vi "运维调试_质控单元.vi"() -> ()   [LabVIEW 2016, in "质控单元.lvlib"]
uses:
  <vilib>/Utility/miscctls.llb/LVPointTypeDef.ctl
  <vilib>/Analysis/6fits.llb/Curve Fitting Criteria.ctl
  <vilib>/Plasmionique/MB Master/MB_Master_Serial/MB_Master_Serial.lvclass
  D:/Program Files (x86)/National Instruments/LabVIEW 2016/vi.lib/Plasmionique/MB Master/MB_Master/MB_Master.lvclass
  <vilib>/Utility/config.llb/Write Key (I32).vi
  <vilib>/Utility/config.llb/Write Key (Double).vi
  <vilib>/Utility/config.llb/Write Key (Boolean).vi
  <vilib>/Utility/config.llb/Write Key (U32).vi
  <vilib>/Utility/config.llb/Read Key (I32).vi
  <vilib>/Utility/config.llb/Read Key (Double).vi
  <vilib>/Utility/config.llb/Read Key (Boolean).vi
  <vilib>/Utility/config.llb/Read Key (U32).vi
  <vilib>/Plasmionique/MB Master/MB Master.lvlib
  <vilib>/ptbypt/NI_PtbyPt.lvlib
  <vilib>/Utility/config.llb/NI_LVConfig.lvlib
  <vilib>/Analysis/NI_AALPro.lvlib
panel:
  out "COM口":string
  in  "总磷模块选择":enum32{"氨氮总磷", "总氮总磷"}(ring)=enum."总氮总磷"
  out "质控流程中":bool
  out "CODMn质控中断报警":bool
  out "总磷质控中断报警":bool
  out "总氮质控中断报警":bool
  out "氨氮质控中断报警":bool
  in  "报警清除":bool
  in  "CODMn量程选择":enum32{"H", "L", "AUTO"}(ring)
  in  "CODMn加标回收启动":bool
  in  "总磷总氮加标回收启动":bool
  in  "氨氮加标回收启动":bool
  in  "总磷量程选择":enum32{"H", "L", "AUTO"}(ring)=enum."AUTO"
  in  "总氮量程选择":enum32{"H", "L", "AUTO"}(ring)=enum."AUTO"
  in  "氨氮量程选择":enum32{"H", "L", "AUTO"}(ring)=enum."AUTO"
  out "COD超时报警":bool
  out "总磷总氮超时报警":bool
  out "氨氮进样超时报警":bool
  out "簇":T1
  out "通讯指示灯3":bool
  out "通讯指示灯2":bool
  out "通讯指示灯1":bool
  in  "CODMn":bool
  in  "总磷总氮":bool
  in  "氨氮":bool
  in  "枚举":enum16{"柱塞泵1", "柱塞泵2", "柱塞泵3"}(ring)
  in  "启用":bool
  in  "B 3":dbl caption="B3"
  in  "K 3":dbl caption="K3"
  in  "B 2":dbl caption="B2"
  in  "K 2":dbl caption="K2"
  in  "B":dbl caption="B1"
  in  "K":dbl caption="K1"
  out "r^2":dbl format="%_6g"
  out "拟合方程":string
  in  "实际体积 5":dbl
  in  "标准体积 5":dbl
  in  "实际体积 4":dbl
  in  "标准体积 4":dbl
  in  "实际体积 3":dbl
  in  "实际体积 2":dbl
  in  "实际体积 1":dbl
  in  "标准体积 3":dbl
  in  "标准体积 2":dbl
  in  "标准体积 1":dbl
  in  "读取":bool
  in  "柱塞泵3":bool
  in  "柱塞泵2":bool
  in  "柱塞泵1":bool
  in  "注出体积选择":u16(ring) items=["0.1mL", "0.3mL", "0.5mL", "0.8mL", "1.0mL"]
  out "Serial Config":T2={"baud rate (bps)"=115200, "stop bits"=10, "parity"=0, "flow control"=0, "timeout"=100, "retries"=1} {"stop bits" items=["1.0"=10, "1.5"=15, "2.0"=20]; "parity" items=["None", "Odd", "Even", "Mark", "Space"]; "flow control" items=["None", "XON/XOFF", "RTS/CTS", "XON/XOFF & RTS/CTS", "DTR/DSR", "XON/XOFF & DTR/DSR"]}
  out "VISA Resource":refnum<visa-resource-name>="COM8"
  in  "背隙补偿步数 3":i32 min=0 max=2000
  in  "背隙补偿步数 2":i32 min=0 max=2000
  in  "写入":bool
  in  "背隙补偿步数":i32 min=0 max=2000
  out "启动模块":T3
  out "COD传感器故障报警":bool
  in  "总氮停止":bool
  in  "总氮排液":bool
  in  "总氮调试":bool
  out "总氮加标回收率":dbl caption="加标回收率" format="%.2f"
  out "总氮加标体积":dbl caption="加标体积" format="%.3f"
  out "总氮母液浓度":dbl caption="加标母液浓度" format="%.3f"
  out "总氮加标水杯定容体积":dbl caption="加标水杯定容体积" format="%.2f"
  out "总氮加标后水样浓度":dbl caption="加标后水样浓度" format="%.3f"
  out "总氮加标前水样浓度":dbl caption="加标前水样浓度" format="%.3f"
  out "总氮检出限":dbl caption="检出限" format="%.3f"
  out "总氮量程":dbl caption="量程" format="%.2f"
  out "总氮状态":u16(ring) caption="状态" items=["待机", "润洗", "进样", "等待取液", "排液"]
  in  "返回":bool
  in  "查看":bool
  out "直接启动":bool
  out "常规启动":bool
  out "总磷总氮传感器故障报警":bool
  out "氨氮传感器故障报警":bool
  out "columns":string[](array[string])
  out "data":T4
  out "COD平行样测完标志":bool
  out "氨氮总磷平行样测完标志":bool
  out "输出簇 2":T5
  out "常规启动 2":bool
  out "直接启动 2":bool
  out "启动模块 2":cluster{"氨氮1":bool, "总磷1":bool, " COD1":bool}
  in  "停止测量":bool
  out "输出簇":T6
  in  "加标回收":bool
  in  "平行样测试":bool
  in  "CODMn停止":bool
  in  "CODMn排液":bool
  in  "CODMn调试":bool
  in  "总磷停止":bool
  in  "总磷排液":bool
  in  "总磷调试":bool
  out "COD加标回收率":dbl caption="加标回收率" format="%.2f"
  out "COD加标体积":dbl caption="加标体积" format="%.3f"
  out "COD母液浓度":dbl caption="加标母液浓度" format="%.2f"
  out "COD加标水杯定容体积":dbl caption="加标水杯定容体积" format="%.2f"
  out "COD加标后水样浓度":dbl caption="加标后水样浓度" format="%.2f"
  out "COD加标前水样浓度":dbl caption="加标前水样浓度" format="%.2f"
  out "COD检出限":dbl caption="检出限" format="%.2f"
  out "COD量程":dbl caption="量程" format="%.2f"
  out "COD状态":u16(ring) caption="状态" items=["待机", "润洗", "进样", "等待取液", "排液"]
  out "总磷加标回收率":dbl caption="加标回收率" format="%.2f"
  out "总磷加标体积":dbl caption="加标体积" format="%.3f"
  out "总磷母液浓度":dbl caption="加标母液浓度" format="%.3f"
  out "总磷加标水杯定容体积":dbl caption="加标水杯定容体积" format="%.2f"
  out "总磷加标后水样浓度":dbl caption="加标后水样浓度" format="%.3f"
  out "总磷加标前水样浓度":dbl caption="加标前水样浓度" format="%.3f"
  out "总磷检出限":dbl caption="检出限" format="%.3f"
  out "总磷量程":dbl caption="量程" format="%.2f"
  out "总磷状态":u16(ring) caption="状态" items=["待机", "润洗", "进样", "等待取液", "排液"]
  out "氨氮加标回收率":dbl caption="加标回收率" format="%.2f"
  out "氨氮加标体积":dbl caption="加标体积" format="%.3f"
  out "氨氮母液浓度":dbl caption="加标母液浓度" format="%.3f"
  out "氨氮加标水杯定容体积":dbl caption="加标水杯定容体积" format="%.2f"
  out "氨氮加标后水样浓度":dbl caption="加标后水样浓度" format="%.3f"
  out "氨氮加标前水样浓度":dbl caption="加标前水样浓度" format="%.3f"
  out "氨氮检出限":dbl caption="检出限" format="%.3f"
  out "氨氮量程":dbl caption="量程" format="%.2f"
  out "氨氮状态":u16(ring) caption="状态" items=["待机", "润洗", "进样", "等待取液", "排液"]
  in  "氨氮停止":bool
  in  "氨氮排液":bool
  in  "氨氮调试":bool
  # "参数配置区"
  # "2000步等于1mL\n100步等于0.05mL\n20步等于0.01mL\n2步等于0.001mL\n（初始默认100步）"
  # "辅助计算区"
  # "状态显示区"
  # "总氮质控参数"
  # "%"
  # "mL"
  # "mg/L"
  # "mL"
  # "mg/L"
  # "mg/L"
  # "mg/L"
  # "mg/L"
  # "CODMn质控参数"
  # "%"
  # "mL"
  # "mg/L"
  # "mL"
  # "mg/L"
  # "mg/L"
  # "mg/L"
  # "mg/L"
  # "总磷质控参数"
  # "%"
  # "mL"
  # "mg/L"
  # "mL"
  # "mg/L"
  # "mg/L"
  # "mg/L"
  # "mg/L"
  # "氨氮质控参数"
  # "%"
  # "mL"
  # "mg/L"
  # "mL"
  # "mg/L"
  # "mg/L"
  # "mg/L"
  # "mg/L"
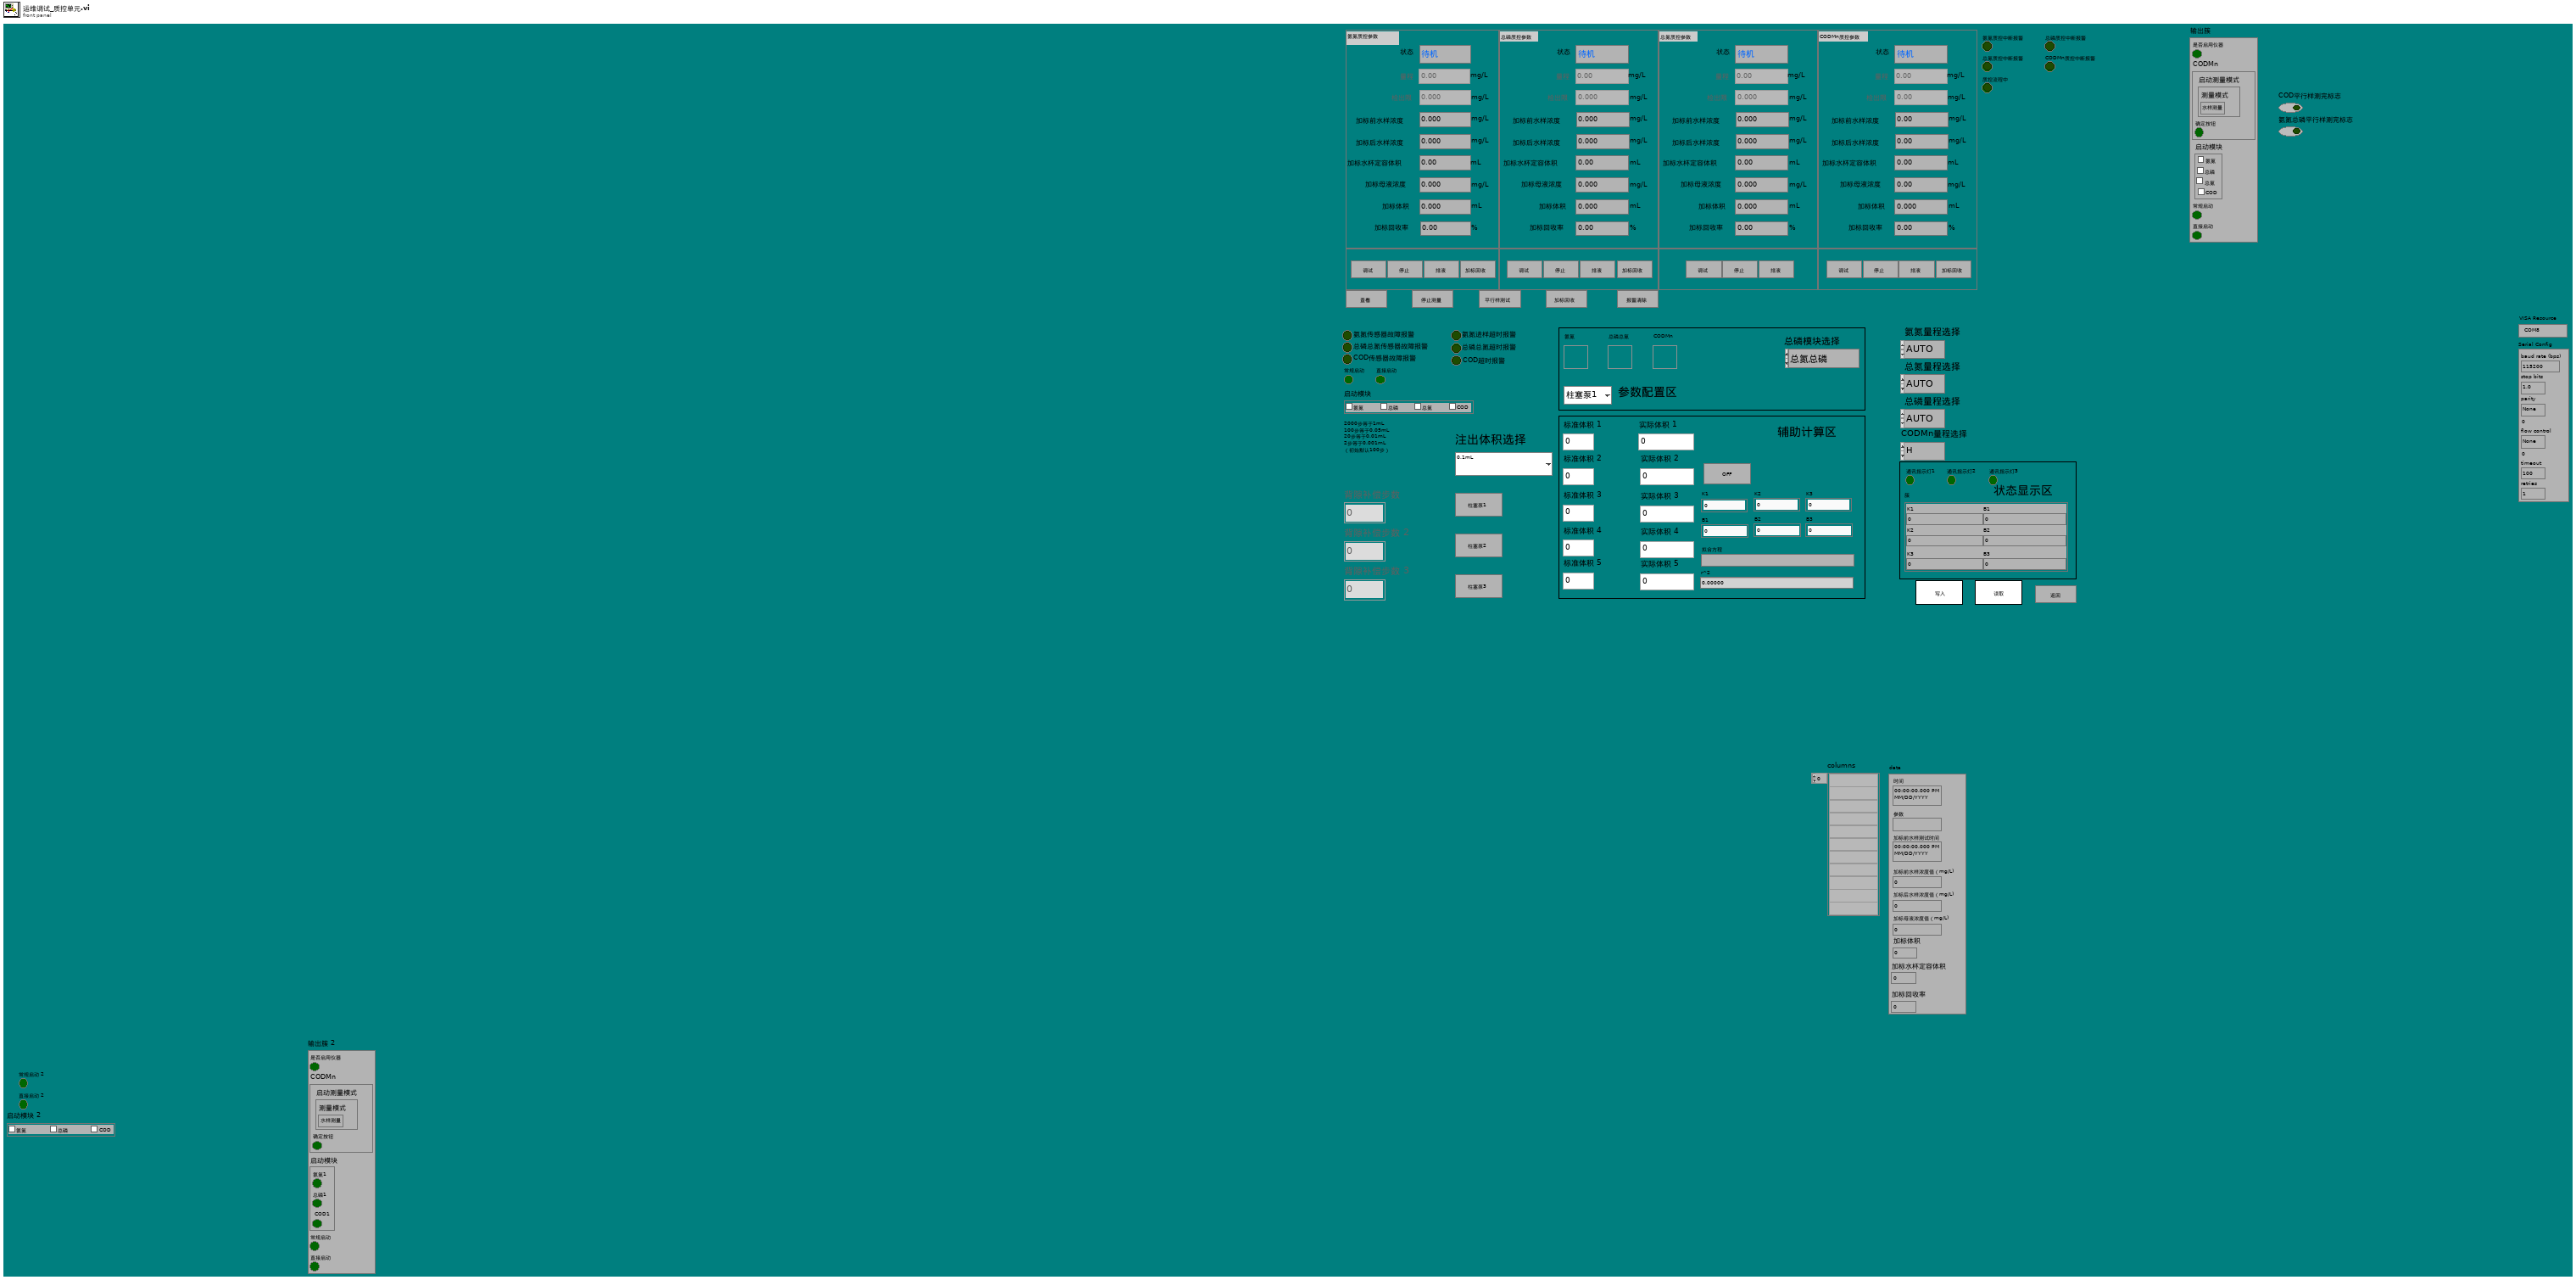
[diagram p1: front panel]
types:
  T1 = cluster{"K1":sgl, "B1":sgl, "K2":sgl, "B2":sgl, "K3":sgl, "B3":sgl}
  T2 = cluster{"baud rate (bps)":u32, "stop bits":u16, "parity":u16, "flow control":u16, "timeout":u32, "retries":i32}
  T3 = cluster{"氨氮":bool, "总磷":bool, "总氮":bool, "COD":bool}
  T4 = cluster{"时间":timestamp, "参数":string, "加标前水样测试时间":timestamp, "加标前水样浓度值（mg/L)":sgl, "加标后水样浓度值（mg/L)":sgl, "加标母液浓度值（mg/L)":sgl, "加标体积":dbl, "加标水杯定容体积":dbl, "加标回收率":dbl}
  T5 = cluster{"是否启用仪器":bool, "CODMn":cluster{"启动测量模式":cluster{"测量模式":enum16{"水样测量", "标样核查", "加标回收", "平行样", "校零", "校标"}}, "确定按钮":bool}, "启动模块":cluster{"氨氮1":bool, "总磷1":bool, " COD1":bool}, "常规启动":bool, "直接启动":bool}
  T6 = cluster{"是否启用仪器":bool, "CODMn":cluster{"启动测量模式":cluster{"测量模式":enum16{"水样测量", "标样核查", "加标回收", "平行样", "校零", "校标"}}, "确定按钮":bool}, "启动模块 3":cluster{"氨氮":bool, "总磷":bool, "总氮":bool, "COD":bool}, "常规启动":bool, "直接启动":bool}
  T7 = typedef "LVPointTypeDef.ctl" = cluster{"Horizontal":i16, "Vertical":i16}
  T8 = cluster{"量程":dbl, "检出限":dbl, "加标前水样浓度":dbl, "加标后水样浓度":dbl, "加标水杯定容体积":dbl, "加标母液浓度":dbl, "加标体积":dbl, "加标回收率":dbl}
  T9 = cluster{"因子编码":u32, "单位":u16, "标样参考值":sgl, "水样数据时间":timestamp, "水样实测值":sgl, "水样数据标识":string, "标样数据时间":timestamp, "标样实测值":sgl, "标样数据标识":string, "空白数据时间":timestamp, "空白实测值":sgl, "空白数据标识":string, "零点核查数据时间":timestamp, "零点核查实测值":sgl, "零点核查数据标识":string, "跨度核查数据时间":timestamp, "跨度核查实测值":sgl, "跨度核查数据标识":string, "加标回收数据时间":timestamp, "加标回收实测值":sgl, "加标回收数据标识":string, "平行样数据时间":timestamp, "平行样实测值":sgl, "平行样数据标识":string}
  T10 = cluster{"因子编码":u32, "单位":u16, "标样参考值":sgl, "水样数据时间":timestamp, "水样实测值":sgl, "水样数据标识":string, "标样数据时间":timestamp, "标样实测值":sgl, "标样数据标识":string, "空白数据时间":timestamp, "空白实测值":sgl, "空白数据标识":string, "零点核查数据时间":timestamp, "零点核查实测值":sgl, "零点核查数据标识":string, "跨度核查数据时间":timestamp, "跨度核查实测值":sgl, "跨度核查数据标识":string, "加标回收数据时间":timestamp, "加标回收实测值":sgl, "加标回收数据标识":string, "平行样数据时间":timestamp, "平行样实测值":sgl, "平行样数据标识":string, "F0":sgl, "F1":sgl, "F2":sgl, "F3":sgl, "F4":sgl, "F5":sgl, "F6":sgl, "F7":sgl, "温度":sgl, "湿度":sgl, "X值":sgl}
  T11 = enum8{"Enabled", "Disabled", "Disabled and Grayed Out"}
  T12 = typedef "NI_AALPro.lvlib/Curve Fitting Criteria.ctl" = u16
  T13 = typedef "NI_LVConfig.lvlib/Config Data RefNum.ctl" = refnum<k1>
  T14 = cluster{"是否启用仪器":bool, "CODMn":cluster{"启动测量模式":cluster{"测量模式":enum16{"水样测量", "标样核查", "加标回收", "平行样", "校零", "校标"}}, "确定按钮":bool}, "启动模块":cluster{"氨氮":bool, "总磷":bool, "总氮":bool, "COD":bool}, "常规启动":bool, "直接启动":bool}
  T15 = cluster{"命令":string, cluster{"starting address":u16, "holding register value":u16}}
  T16 = enum32{"Bad", "Idle", "Run top level", "Running"}
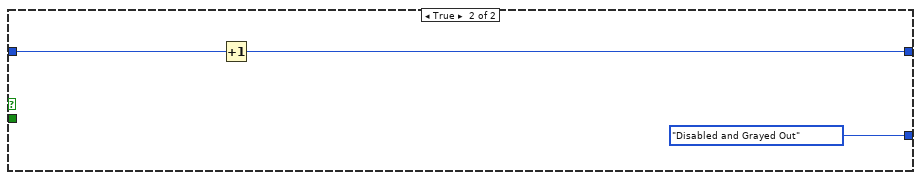
[diagram p3: hidden frame]
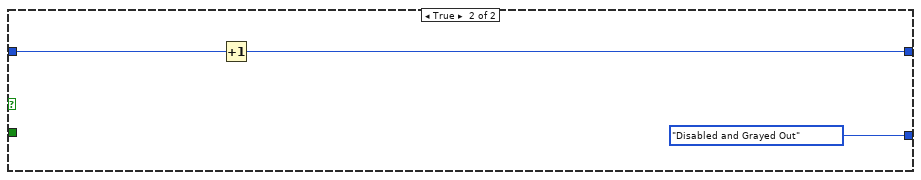
[diagram p5: hidden frame]
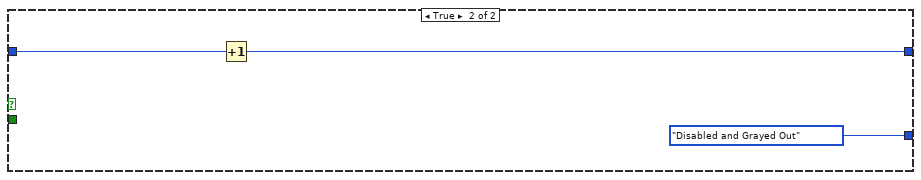
[diagram p7: hidden frame]
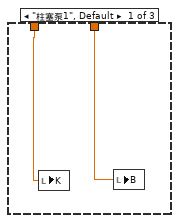
[diagram p9: hidden frame]
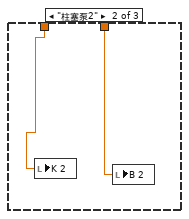
[diagram p10: hidden frame]
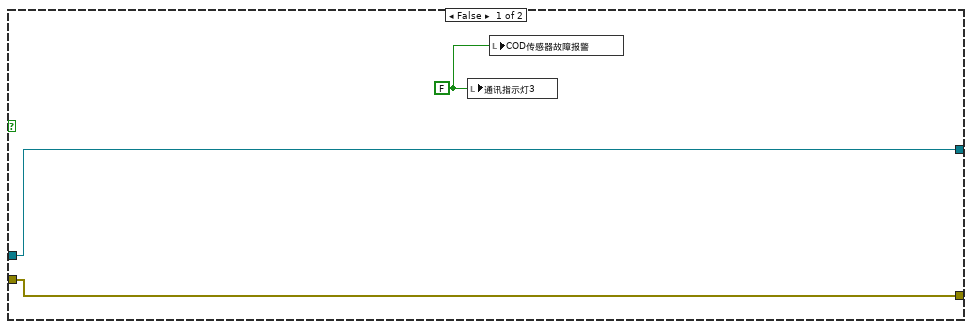
[diagram p11: hidden frame]
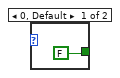
[diagram p12: hidden frame]
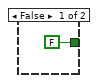
[diagram p13: hidden frame]
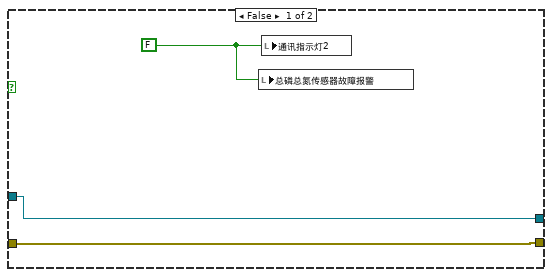
[diagram p14: hidden frame]
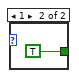
[diagram p16: hidden frame]
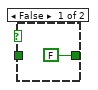
[diagram p17: hidden frame]
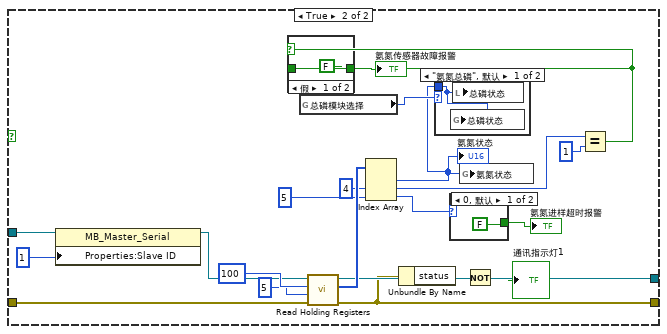
[diagram p18: hidden frame]
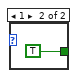
[diagram p20: hidden frame]
diagram:
  w28 = "质控模块量程选择" ("section")
  w7 = "质控模块选择" ("section")
  w78 = "质控线性参数" ("section")
  w96 = "质控背隙补偿" ("section")
  w103 = T2 {"baud rate (bps)"=115200, "stop bits"=10, "parity"=0, "flow control"=0, "timeout"=500, "retries"=1} ("Serial Config")
  w4 = refnum<visa-resource-name> "COM8" ("VISA Resource")
  n1 = global write "串口参数全局.vi" "Serial Config"(w103) -> ()
  n2 = control-ref of="总氮加标回收率"() -> (w120:refnum<vi>)
  n3 = control-ref of="总氮加标体积"() -> (w121:refnum<vi>)
  n4 = control-ref of="总氮加标水杯定容体积"() -> (w123:refnum<vi>)
  n5 = control-ref of="总氮加标后水样浓度"() -> (w124:refnum<vi>)
  n6 = control-ref of="总氮母液浓度"() -> (w122:refnum<vi>)
  n7 = control-ref of="总氮检出限"() -> (w126:refnum<vi>)
  n8 = control-ref of="总氮加标前水样浓度"() -> (w125:refnum<vi>)
  n9 = global write "串口参数全局.vi" "VISA Resource"(w4) -> ()
  n10 = control-ref of="总氮量程"() -> (w127:refnum<vi>)
  n11 = call <vilib>:"Open Serial Session.vi"("Mode (RTU)"=enum16{"RTU", "ASCII"}."RTU", "Slave ID"=u8 10, "Serial Config"=w103, "VISA Resource"=w4) -> ("Error out"=w145:errorcluster, "MB_Serial session"=w146:refnum<class "MB_Master_Serial.lvclass">)  [unwired: 6 in]
  n12 = control-ref of="COD加标水杯定容体积"() -> (w151:refnum<vi>)
  n13 = control-ref of="COD加标前水样浓度"() -> (w153:refnum<vi>)
  n14 = control-ref of="COD加标后水样浓度"() -> (w152:refnum<vi>)
  n15 = property on="窗格" class="Pane"("Origin"=T7 {"Horizontal"=0, "Vertical"=0} ("原点")) -> ()  [unwired: 2 in, 2 out]
  n16 = property on="窗格" class="Pane"("Origin"=T7 {"Horizontal"=0, "Vertical"=0} ("原点")) -> ()  [unwired: 2 in, 2 out]
  n17 = call "质控参数读取.vi"("section"="氨氮质控参数") -> ("error out"=w176:errorcluster, "参数"=w195:T8)  [unwired: 9 in]
  n18 = while {
    tunnel: w146 -> [w244]
    tunnel: w145 -> [w243]
    tunnel: [w210] -> w144
    tunnel: [w219] -> w104
    stop <- FALSE stop-if-true
    n19 = local read "氨氮"() -> (w209:bool)
    n20 = case shown="假" w209 {
      tunnel: w244 -> [w303 w324]
      tunnel: w243 -> [w302 w323]
      tunnel: [w303 w312] -> w214
      tunnel: [w302 w311] -> w212
      frame False {
        w301 = FALSE ("通讯指示灯1")
        n21 = local write "通讯指示灯1"(w301) -> ()
        n22 = local write "氨氮传感器故障报警"(w301) -> ()
      }
      frame True {
        n23 = property class="MB_Master_Serial"(reference=w324, "Properties:Slave ID"=u8 1 ("Slave ID")) -> (reference out=w319:refnum<class "MB_Master_Serial.lvclass">)  [unwired: 1 in, 1 out]
        n24 = global read "质控测完标志全局 1.vi" "总磷模块选择"() -> (w305:enum32{"氨氮总磷", "总氮总磷"})
        n25 = call <vilib>:"Read Holding Registers.vi"("error in (no error)"=w323, "quantity"=u16 5, "starting address"=u16 100, "MB session in"=w319) -> ("error out"=w311:errorcluster, "Registers"=w320:u16[], "MB session out"=w312:refnum<class "MB_Master_Serial.lvclass">)  [unwired: 5 in]
        n26 = Index Array(array=w320, index #2=4 ("索引"), index #3=5 ("索引")) -> (element #1=w304:u16, element #2=w316:u16, element #3=w307:u16)  [unwired: 1 in]
        "氨氮状态" <- w304
        n27 = Unbundle By Name(w311) -> ("status"=w310:bool)
        n28 = case shown="\"氨氮总磷\", 默认" w305 {
          tunnel: w304 -> [w325 _]
          frame "氨氮总磷", Default {
            n29 = global write "氨氮加标回收状态全局变量.vi" "总磷状态"(w325) -> ()
            n30 = local write "总磷状态"(w325) -> ()
          }
          frame "总氮总磷" {
          }
        }
        n31 = case shown="0, 默认" w307 {
          tunnel: [FALSE TRUE] -> w306
          frame 0, Default {
          }
          frame 1 {
          }
        }
        "氨氮进样超时报警" <- w306
        n32 = global write "氨氮加标回收状态全局变量.vi" "氨氮状态"(w304) -> ()
        n33 = Not(x=w310) -> (.not. x?=→"通讯指示灯1":bool)
        n34 = Equal?(x=w316, y=u16 1) -> (x = y?=w313:bool)
        n35 = case shown="假" w313 {
          tunnel: w313 -> [_ w329]
          tunnel: [FALSE w329] -> w314
          frame False {
          }
          frame True {
          }
        }
        "氨氮传感器故障报警" <- w314
      }
    }
    n36 = global read "质控测完标志全局 1.vi" "总磷总氮平行样测完标志"() -> (→"氨氮总磷平行样测完标志":bool)
    n37 = global read "质控测完标志全局 1.vi" "COD加标回收测完标志"() -> (w225:bool)
    n38 = global read "质控测完标志全局 1.vi" "氨氮加标回收测完标志"() -> (w230:bool)
    n39 = global read "质控测完标志全局 1.vi" "总磷加标回收测完标志"() -> (w218:bool)
    n40 = global read "质控测完标志全局 1.vi" "总氮加标回收测完标志"() -> (w216:bool)
    n41 = global read "质控测完标志全局 1.vi" "COD平行样测完标志"() -> (→"COD平行样测完标志":bool)
    n42 = global read "水样浓度全局.vi" "COD加标前水样浓度"() -> (w238:dbl)
    n43 = local read "总氮加标前水样浓度"() -> (w222:dbl)
    n44 = global read "水样浓度全局.vi" "氨氮加标前水样浓度"() -> (w242:dbl)
    n45 = global read "水样浓度全局.vi" "总磷加标前水样浓度"() -> (w240:dbl)
    n46 = local read "COD加标前水样浓度"() -> (w237:dbl)
    n47 = global read "水样浓度全局.vi" "总氮加标前水样浓度"() -> (w221:dbl)
    n48 = local read "氨氮加标前水样浓度"() -> (w241:dbl)
    n49 = local read "总磷加标前水样浓度"() -> (w239:dbl)
    n50 = Wait (ms)(milliseconds to wait=u32 1000 ("等待时间（毫秒）")) -> ()  [unwired: 1 out]
    n51 = Not Equal?(x=w242, y=w241) -> (x != y?=w236:bool)
    n52 = Not Equal?(x=w240, y=w239) -> (x != y?=w234:bool)
    n53 = Not Equal?(x=w238, y=w237) -> (x != y?=w233:bool)
    n54 = Not Equal?(x=w221, y=w222) -> (x != y?=w220:bool)
    n55 = call <vilib>:"Boolean Crossing PtByPt.vi"("direction"=enum16{"either", "false-true", "true-false"}."false-true", "input"=w230) -> ("crossing"=w229:bool)  [unwired: 1 in]
    n56 = call <vilib>:"Boolean Crossing PtByPt.vi"("direction"=enum16{"either", "false-true", "true-false"}."false-true", "input"=w218) -> ("crossing"=w226:bool)  [unwired: 1 in]
    n57 = call <vilib>:"Boolean Crossing PtByPt.vi"("direction"=enum16{"either", "false-true", "true-false"}."false-true", "input"=w225) -> ("crossing"=w223:bool)  [unwired: 1 in]
    n58 = call <vilib>:"Boolean Crossing PtByPt.vi"("direction"=enum16{"either", "false-true", "true-false"}."false-true", "input"=w216) -> ("crossing"=w215:bool)  [unwired: 1 in]
    n59 = case shown="真" w229 {
      frame False {
      }
      frame True {
        n60 = flat-sequence {
          frame #0 {
            n61 = global read "VAR总磷氨氮全局变量.vi" "测量数据区"() -> (w383:T9)
            n62 = Unbundle By Name(w383) -> ("加标回收实测值"=w384:sgl)
            n63 = property on="氨氮加标后水样浓度" class="DigNum (严格)"("Val(Sgnl)"=w384) -> ()  [unwired: 2 in, 2 out]
          }
          frame #1 {
            n64 = Wait (ms)(milliseconds to wait=u32 500 ("等待时间（毫秒）")) -> ()  [unwired: 1 out]
          }
          frame #2 {
            n65 = global read "VAR总磷氨氮全局变量.vi" "测量数据区"() -> (w388:T9)
            n66 = global read "VAR总磷氨氮全局变量.vi" "测量数据区"() -> (w387:T9)
            n67 = global read "VAR总磷氨氮全局变量.vi" "测量数据区"() -> (w386:T9)
            n68 = local read "氨氮加标水杯定容体积"() -> (w395:dbl)
            n69 = global read "水样浓度全局.vi" "氨氮加标前水样浓度"() -> (w399:dbl)
            n70 = Unbundle By Name(w388) -> ("加标回收数据时间"=w392:timestamp)
            n71 = Unbundle By Name(w386) -> ("加标回收实测值"=w398:sgl)
            n72 = Unbundle By Name(w387) -> ("水样数据时间"=w390:timestamp)
            n73 = local read "氨氮加标回收率"() -> (w394:dbl)
            n74 = local read "氨氮母液浓度"() -> (w397:dbl)
            n75 = local read "氨氮加标体积"() -> (w396:dbl)
            n76 = Bundle By Name(cluster=T4 {"时间"=timestamp(0 s since 1904-01-01), "参数"="", "加标前水样测试时间"=timestamp(0 s since 1904-01-01), "加标前水样浓度值（mg/L)"=0.0, "加标后水样浓度值（mg/L)"=0.0, "加标母液浓度值（mg/L)"=0.0, "加标体积"=0.0, "加标水杯定容体积"=0.0, "加标回收率"=0.0} ("data"), "时间"=w392, "参数"="氨氮加标回收率" ("table"), "加标前水样测试时间"=w390, "加标前水样浓度值（mg/L)"=w399, "加标后水样浓度值（mg/L)"=w398, "加标母液浓度值（mg/L)"=w397, "加标体积"=w396, "加标水杯定容体积"=w395, "加标回收率"=w394) -> (w389:T4)
            n77 = local read "columns"() -> (w400:string[])
            n78 = call "数据写入database.vi"("data"=w389, "columns"=w400, "table"="加标回收率") -> ()  [unwired: 8 in, 1 out]
            n79 = local write "data"(w389) -> ()
          }
        }
      }
    }
    n80 = case shown="真" w226 {
      frame False {
      }
      frame True {
        n81 = flat-sequence {
          frame #0 {
            n82 = global read "VAR总磷氨氮全局变量.vi" "总磷测量数据区"() -> (w365:T10)
            n83 = Unbundle By Name(w365) -> ("加标回收实测值"=w364:sgl)
            n84 = property on="总磷加标后水样浓度" class="DigNum (严格)"("Val(Sgnl)"=w364) -> ()  [unwired: 2 in, 2 out]
          }
          frame #1 {
            n85 = Wait (ms)(milliseconds to wait=u32 500 ("等待时间（毫秒）")) -> ()  [unwired: 1 out]
          }
          frame #2 {
            n86 = global read "VAR总磷氨氮全局变量.vi" "总磷测量数据区"() -> (w372:T10)
            n87 = global read "VAR总磷氨氮全局变量.vi" "总磷测量数据区"() -> (w368:T10)
            n88 = global read "VAR总磷氨氮全局变量.vi" "总磷测量数据区"() -> (w379:T10)
            n89 = local read "总磷加标水杯定容体积"() -> (w375:dbl)
            n90 = global read "水样浓度全局.vi" "总磷加标前水样浓度"() -> (w380:dbl)
            n91 = Unbundle By Name(w372) -> ("加标回收数据时间"=w369:timestamp)
            n92 = Unbundle By Name(w379) -> ("加标回收实测值"=w378:sgl)
            n93 = Unbundle By Name(w368) -> ("水样数据时间"=w367:timestamp)
            n94 = local read "总磷加标回收率"() -> (w374:dbl)
            n95 = local read "总磷母液浓度"() -> (w377:dbl)
            n96 = local read "总磷加标体积"() -> (w376:dbl)
            n97 = Bundle By Name(cluster=T4 {"时间"=timestamp(0 s since 1904-01-01), "参数"="", "加标前水样测试时间"=timestamp(0 s since 1904-01-01), "加标前水样浓度值（mg/L)"=0.0, "加标后水样浓度值（mg/L)"=0.0, "加标母液浓度值（mg/L)"=0.0, "加标体积"=0.0, "加标水杯定容体积"=0.0, "加标回收率"=0.0} ("data"), "时间"=w369, "参数"="总磷加标回收率" ("table"), "加标前水样测试时间"=w367, "加标前水样浓度值（mg/L)"=w380, "加标后水样浓度值（mg/L)"=w378, "加标母液浓度值（mg/L)"=w377, "加标体积"=w376, "加标水杯定容体积"=w375, "加标回收率"=w374) -> (w373:T4)
            "data" <- w373
            n98 = local read "columns"() -> (w381:string[])
            n99 = call "数据写入database.vi"("data"=w373, "columns"=w381, "table"="加标回收率") -> ()  [unwired: 8 in, 1 out]
          }
        }
      }
    }
    n100 = case shown="真" w223 {
      frame False {
      }
      frame True {
        n101 = flat-sequence {
          frame #0 {
            n102 = global read "COD浓度全局变量.vi" "COD浓度（mg/L)"() -> (w349:dbl)
            n103 = property on="COD加标后水样浓度" class="DigNum (严格)"("Val(Sgnl)"=w349) -> ()  [unwired: 2 in, 2 out]
          }
          frame #1 {
            n104 = Wait (ms)(milliseconds to wait=u32 500 ("等待时间（毫秒）")) -> ()  [unwired: 1 out]
          }
          frame #2 {
            n105 = local read "COD加标水杯定容体积"() -> (w357:dbl)
            n106 = global read "水样浓度全局.vi" "COD加标前水样浓度"() -> (w361:dbl)
            n107 = global read "COD浓度全局变量.vi" "COD浓度（mg/L)"() -> (w360:dbl)
            n108 = global read "COD测量模式全局.vi" "加标回收启动时间"() -> (w352:timestamp)
            n109 = global read "COD测量模式全局.vi" "水样启动时间"() -> (w351:timestamp)
            n110 = local read "COD加标回收率"() -> (w356:dbl)
            n111 = local read "COD母液浓度"() -> (w359:dbl)
            n112 = local read "COD加标体积"() -> (w358:dbl)
            n113 = Bundle By Name(cluster=T4 {"时间"=timestamp(0 s since 1904-01-01), "参数"="", "加标前水样测试时间"=timestamp(0 s since 1904-01-01), "加标前水样浓度值（mg/L)"=0.0, "加标后水样浓度值（mg/L)"=0.0, "加标母液浓度值（mg/L)"=0.0, "加标体积"=0.0, "加标水杯定容体积"=0.0, "加标回收率"=0.0} ("data"), "时间"=w352, "参数"="CODMn加标回收率" ("table"), "加标前水样测试时间"=w351, "加标前水样浓度值（mg/L)"=w361, "加标后水样浓度值（mg/L)"=w360, "加标母液浓度值（mg/L)"=w359, "加标体积"=w358, "加标水杯定容体积"=w357, "加标回收率"=w356) -> (w355:T4)
            n114 = local read "columns"() -> (w362:string[])
            n115 = call "数据写入database.vi"("data"=w355, "columns"=w362, "table"="加标回收率") -> ()  [unwired: 8 in, 1 out]
            n116 = local write "data"(w355) -> ()
          }
        }
      }
    }
    n117 = case shown="真" w215 {
      frame False {
      }
      frame True {
        n118 = flat-sequence {
          frame #0 {
            n119 = global read "VAR总氮全局变量.vi" "总氮测量数据区"() -> (w330:T10)
            n120 = Unbundle By Name(w330) -> ("加标回收实测值"=w331:sgl)
            n121 = property on="总氮加标后水样浓度" class="DigNum (严格)"("Val(Sgnl)"=w331) -> ()  [unwired: 2 in, 2 out]
          }
          frame #1 {
            n122 = Wait (ms)(milliseconds to wait=u32 500 ("等待时间（毫秒）")) -> ()  [unwired: 1 out]
          }
          frame #2 {
            n123 = global read "VAR总氮全局变量.vi" "总氮测量数据区"() -> (w334:T10)
            n124 = global read "VAR总氮全局变量.vi" "总氮测量数据区"() -> (w335:T10)
            n125 = global read "VAR总氮全局变量.vi" "总氮测量数据区"() -> (w333:T10)
            n126 = local read "总氮加标水杯定容体积"() -> (w342:dbl)
            n127 = global read "水样浓度全局.vi" "总氮加标前水样浓度"() -> (w346:dbl)
            n128 = Unbundle By Name(w335) -> ("加标回收数据时间"=w338:timestamp)
            n129 = Unbundle By Name(w333) -> ("加标回收实测值"=w345:sgl)
            n130 = Unbundle By Name(w334) -> ("水样数据时间"=w337:timestamp)
            n131 = local read "总氮加标回收率"() -> (w341:dbl)
            n132 = local read "总氮母液浓度"() -> (w344:dbl)
            n133 = local read "总氮加标体积"() -> (w343:dbl)
            n134 = Bundle By Name(cluster=T4 {"时间"=timestamp(0 s since 1904-01-01), "参数"="", "加标前水样测试时间"=timestamp(0 s since 1904-01-01), "加标前水样浓度值（mg/L)"=0.0, "加标后水样浓度值（mg/L)"=0.0, "加标母液浓度值（mg/L)"=0.0, "加标体积"=0.0, "加标水杯定容体积"=0.0, "加标回收率"=0.0} ("data"), "时间"=w338, "参数"="总氮加标回收率" ("table"), "加标前水样测试时间"=w337, "加标前水样浓度值（mg/L)"=w346, "加标后水样浓度值（mg/L)"=w345, "加标母液浓度值（mg/L)"=w344, "加标体积"=w343, "加标水杯定容体积"=w342, "加标回收率"=w341) -> (w336:T4)
            n135 = local read "columns"() -> (w347:string[])
            n136 = call "数据写入database.vi"("data"=w336, "columns"=w347, "table"="加标回收率") -> ()  [unwired: 8 in, 1 out]
            n137 = local write "data"(w336) -> ()
          }
        }
      }
    }
    n138 = Compound Arithmetic op=OR ("复合运算")(w236, w234, w233, w220) -> (w235:bool)
    n139 = case shown="真" w235 {
      frame False {
      }
      frame True {
        n140 = global read "水样浓度全局.vi" "COD加标前水样浓度"() -> (w403:dbl)
        n141 = global read "水样浓度全局.vi" "总氮加标前水样浓度"() -> (w402:dbl)
        n142 = global read "水样浓度全局.vi" "总磷加标前水样浓度"() -> (w404:dbl)
        n143 = global read "水样浓度全局.vi" "氨氮加标前水样浓度"() -> (w405:dbl)
        n144 = property on="总氮加标前水样浓度" class="DigNum (严格)"("Val(Sgnl)"=w402) -> ()  [unwired: 2 in, 2 out]
        n145 = property on="COD加标前水样浓度" class="DigNum (严格)"("Val(Sgnl)"=w403) -> ()  [unwired: 2 in, 2 out]
        n146 = property on="总磷加标前水样浓度" class="DigNum (严格)"("Val(Sgnl)"=w404) -> ()  [unwired: 2 in, 2 out]
        n147 = property on="氨氮加标前水样浓度" class="DigNum (严格)"("Val(Sgnl)"=w405) -> ()  [unwired: 2 in, 2 out]
      }
    }
    n148 = local read "总磷总氮"() -> (w208:bool)
    n149 = case shown="真" w208 {
      tunnel: w214 -> [w275 w290]
      tunnel: [w275 w289] -> w213
      tunnel: w212 -> [w274 w288]
      tunnel: [w274 w286] -> w211
      frame False {
        w273 = FALSE ("通讯指示灯2")
        n150 = local write "总磷总氮传感器故障报警"(w273) -> ()
        n151 = local write "通讯指示灯2"(w273) -> ()
      }
      frame True {
        n152 = property class="MB_Master_Serial"(reference=w290, "Properties:Slave ID"=u8 2 ("Slave ID")) -> (reference out=w292:refnum<class "MB_Master_Serial.lvclass">)  [unwired: 1 in, 1 out]
        n153 = global read "质控测完标志全局 1.vi" "总磷模块选择"() -> (w276:enum32{"氨氮总磷", "总氮总磷"})
        n154 = call <vilib>:"Read Holding Registers.vi"("error in (no error)"=w288, "quantity"=u16 5, "starting address"=u16 100, "MB session in"=w292) -> ("error out"=w286:errorcluster, "Registers"=w295:u16[], "MB session out"=w289:refnum<class "MB_Master_Serial.lvclass">)  [unwired: 5 in]
        n155 = Unbundle By Name(w286) -> ("status"=w287:bool)
        n156 = Index Array(array=w295, index #2=4 ("索引")) -> (element #1=w279:u16, element #2=w282:u16, element #3=w277:u16)  [unwired: 2 in]
        "总氮状态" <- w279
        n157 = case shown="0, 默认" w277 {
          tunnel: [FALSE TRUE] -> w278
          frame 0, Default {
          }
          frame 1 {
          }
        }
        "总磷总氮超时报警" <- w278
        n158 = Not(x=w287) -> (.not. x?=→"通讯指示灯2":bool)
        n159 = Equal?(x=w282, y=u16 1) -> (x = y?=w280:bool)
        n160 = case shown="真" w280 {
          tunnel: w280 -> [_ w300]
          tunnel: [FALSE w300] -> w281
          frame False {
          }
          frame True {
          }
        }
        "总磷总氮传感器故障报警" <- w281
        n161 = case shown="\"总氮总磷\"" w276 {
          tunnel: w279 -> [_ w296]
          frame "氨氮总磷", Default {
          }
          frame "总氮总磷" {
            n162 = global write "氨氮加标回收状态全局变量.vi" "总磷状态"(w296) -> ()
            "总磷状态" <- w296
          }
        }
        n163 = global write "氨氮加标回收状态全局变量.vi" "总氮状态"(w279) -> ()
      }
    }
    n164 = local read "CODMn"() -> (w207:bool)
    n165 = case shown="真" w207 {
      tunnel: [w249 w264] -> w219
      tunnel: w213 -> [w249 w256]
      tunnel: w211 -> [w248 w255]
      tunnel: [w248 w253] -> w210
      frame False {
        w247 = FALSE ("通讯指示灯3")
        n166 = local write "通讯指示灯3"(w247) -> ()
        n167 = local write "COD传感器故障报警"(w247) -> ()
      }
      frame True {
        n168 = property class="MB_Master_Serial"(reference=w256, "Properties:Slave ID"=u8 3 ("Slave ID")) -> (reference out=w267:refnum<class "MB_Master_Serial.lvclass">)  [unwired: 1 in, 1 out]
        n169 = call <vilib>:"Read Holding Registers.vi"("error in (no error)"=w255, "quantity"=u16 5, "starting address"=u16 100, "MB session in"=w267) -> ("error out"=w253:errorcluster, "Registers"=w263:u16[], "MB session out"=w264:refnum<class "MB_Master_Serial.lvclass">)  [unwired: 5 in]
        n170 = Unbundle By Name(w253) -> ("status"=w254:bool)
        n171 = Index Array(array=w263, index #2=4 ("索引")) -> (element #1=w261:u16, element #2=w258:u16, element #3=w250:u16)  [unwired: 2 in]
        "COD状态" <- w261
        n172 = global write "氨氮加标回收状态全局变量.vi" "COD状态"(w261) -> ()
        n173 = Not(x=w254) -> (.not. x?=→"通讯指示灯3":bool)
        n174 = case shown="1" w250 {
          tunnel: [FALSE TRUE] -> w251
          frame 0, Default {
          }
          frame 1 {
          }
        }
        "COD超时报警" <- w251
        n175 = Equal?(x=w258, y=u16 1) -> (x = y?=w260:bool)
        n176 = case shown="真" w260 {
          tunnel: w260 -> [_ w272]
          tunnel: [FALSE w272] -> w257
          frame False {
          }
          frame True {
          }
        }
        "COD传感器故障报警" <- w257
      }
    }
  }
  n177 = Build Array(w127, w126, w125, w124, w123, w122, w121, w120) -> (w119:refnum<vi>[])
  n178 = while {
    stop <- FALSE stop-if-true
    n179 = global read "质控测完标志全局 1.vi" "氨氮质控流程中"() -> (w416:bool)
    n180 = global read "质控测完标志全局 1.vi" "COD质控流程中"() -> (w408:bool)
    n181 = global read "质控测完标志全局 1.vi" "总氮质控流程中"() -> (w412:bool)
    n182 = global read "质控中断报警全局.vi" "CODMn中断报警"() -> (→"CODMn质控中断报警":bool)
    n183 = global read "质控中断报警全局.vi" "氨氮中断报警"() -> (→"氨氮质控中断报警":bool)
    n184 = global read "质控中断报警全局.vi" "总氮中断报警"() -> (→"总氮质控中断报警":bool)
    n185 = Wait (ms)(milliseconds to wait=u32 100 ("等待时间（毫秒）")) -> ()  [unwired: 1 out]
    n186 = global read "质控中断报警全局.vi" "总磷中断报警"() -> (→"总磷质控中断报警":bool)
    n187 = local read "COD状态"() -> (w434:u16)
    n188 = global read "质控测完标志全局 1.vi" "质控流程中"() -> (w420:bool)
    "质控流程中" <- w420
    n189 = local read "总氮状态"() -> (w432:u16)
    n190 = local read "氨氮状态"() -> (w448:u16)
    n191 = local read "总磷状态"() -> (w439:u16)
    n192 = global write "质控测完标志全局 1.vi" "总磷模块选择"("总磷模块选择") -> ()
    n193 = Not Equal To 0?(x=w432) -> (x != 0?=w431:bool)
    n194 = Not Equal To 0?(x=w448) -> (x != 0?=w447:bool)
    n195 = Not Equal To 0?(x=w439) -> (x != 0?=w441:bool)
    n196 = Not Equal To 0?(x=w434) -> (x != 0?=w438:bool)
    n197 = Select(t=T11."Disabled and Grayed Out" ("禁用"), s=w447, f=T11."Enabled") -> (s? t:f=w444:T11)
    n198 = Select(t=T11."Disabled and Grayed Out" ("禁用"), s=w441, f=T11."Enabled") -> (s? t:f=w440:T11)
    n199 = Select(t=T11."Disabled and Grayed Out" ("禁用"), s=w438, f=T11."Enabled") -> (s? t:f=w435:T11)
    n200 = Select(t=T11."Disabled and Grayed Out" ("禁用"), s=w416, f=T11."Enabled") -> (s? t:f=w414:T11)
    n201 = Select(t=T11."Disabled and Grayed Out" ("禁用"), s=w408, f=T11."Enabled") -> (s? t:f=w406:T11)
    n202 = Select(t=T11."Disabled and Grayed Out" ("禁用"), s=w412, f=T11."Enabled") -> (s? t:f=w410:T11)
    n203 = Select(t=T11."Disabled and Grayed Out" ("禁用"), s=w431, f=T11."Enabled") -> (s? t:f=w428:T11)
    n204 = Select(t=T11."Disabled and Grayed Out" ("禁用"), s=w420, f=T11."Enabled") -> (s? t:f=w419:T11)
    n205 = property on="氨氮加标回收启动" class="Bool"("DisabledEnum"=w414) -> ()  [unwired: 2 in, 2 out]
    n206 = property on="氨氮调试" class="Bool"("DisabledEnum"=w444) -> ()  [unwired: 2 in, 2 out]
    n207 = property on="总磷调试" class="Bool"("DisabledEnum"=w440) -> ()  [unwired: 2 in, 2 out]
    n208 = property on="COD调试" class="Bool"("DisabledEnum"=w435) -> ()  [unwired: 2 in, 2 out]
    n209 = property on="总磷总氮加标回收启动" class="Bool"("DisabledEnum"=w410) -> ()  [unwired: 2 in, 2 out]
    n210 = property on="CODMn加标回收启动" class="Bool"("DisabledEnum"=w406) -> ()  [unwired: 2 in, 2 out]
    n211 = property on="加标回收" class="Bool"("DisabledEnum"=w419) -> ()  [unwired: 2 in, 2 out]
    n212 = property on="总氮调试" class="Bool"("DisabledEnum"=w428) -> ()  [unwired: 2 in, 2 out]
    n213 = property on="总磷模块选择" class="Enum (严格)"("DisabledEnum"=w419) -> ()  [unwired: 2 in, 2 out]
    n214 = case shown="真" "启用" {
      frame False {
      }
      frame True {
        w466 = T12 0 items=["最小二乘", "最小绝对残差", "Bisquare"] ("method")
        n215 = Build Array("标准体积 1", "标准体积 2", "标准体积 3", "标准体积 4", "标准体积 5") -> (w463:dbl[])
        n216 = Build Array("实际体积 1", "实际体积 2", "实际体积 3", "实际体积 4", "实际体积 5") -> (w464:dbl[])
        n217 = call "线性公式质控用.vi"("标液浓度"=w463, "模型"=enum32{"线性", "多项式"}."线性", "监测浓度"=w464, "启用"=bool[] [TRUE, TRUE, TRUE, TRUE, TRUE], "method"=w466) -> ("拟合方程"=→"拟合方程":string, "r^2"=→"r^2":dbl, "slope"=w452:dbl, "intercept"=w451:dbl)  [unwired: 6 in, 1 out]
        n218 = case shown="\"柱塞泵3\"" "枚举" {
          tunnel: w452 -> [w470 w473 w474]
          tunnel: w451 -> [w471 w472 w475]
          frame "柱塞泵1", Default {
            n219 = local write "K"(w470) -> ()
            n220 = local write "B"(w471) -> ()
          }
          frame "柱塞泵2" {
            n221 = local write "K 2"(w473) -> ()
            n222 = local write "B 2"(w472) -> ()
          }
          frame "柱塞泵3" {
            n223 = local write "K 3"(w474) -> ()
            n224 = local write "B 3"(w475) -> ()
          }
        }
      }
    }
  }
  n225 = while {
    shift-right: [w496] -> _
    shift-left: i16 0 -> [w493]
    shift-right: [w488] -> _
    shift-left: i16 0 -> [w489]
    shift-right: [w487] -> _
    shift-left: i16 0 -> [w490]
    stop <- FALSE stop-if-true
    n226 = local read "柱塞泵2"() -> (w477:bool)
    n227 = local read "柱塞泵3"() -> (w476:bool)
    n228 = local read "柱塞泵1"() -> (w478:bool)
    n229 = Less Or Equal?(x=w493, y=i16 30) -> (x <= y?=w491:bool)
    n230 = Less Or Equal?(x=w490, y=i16 30) -> (x <= y?=w481:bool)
    n231 = Less Or Equal?(x=w489, y=i16 30) -> (x <= y?=w486:bool)
    n232 = Wait (ms)(milliseconds to wait=u32 1000 ("等待时间（毫秒）")) -> ()  [unwired: 1 out]
    n233 = And(x=w491, y=w478) -> (x .and. y?=w494:bool)
    n234 = And(x=w481, y=w476) -> (x .and. y?=w483:bool)
    n235 = And(x=w486, y=w477) -> (x .and. y?=w484:bool)
    n236 = case shown="假" w494 {
      tunnel: w493 -> [_ w519]
      tunnel: [i16 0 w518] -> w496
      tunnel: [T11."Enabled" ("禁用") T11."Disabled and Grayed Out" ("禁用")] -> w495
      tunnel: w478 -> [w513 _]
      frame False {
        n237 = case shown="真" w513 {
          frame False {
          }
          frame True {
            n238 = property on="柱塞泵1" class="Bool (严格)"("Val(Sgnl)"=FALSE ("值(信号)")) -> ()  [unwired: 2 in, 2 out]
          }
        }
      }
      frame True {
        n239 = Increment(x=w519) -> (x+1=w518:i16)
      }
    }
    n240 = case shown="假" w483 {
      tunnel: w490 -> [_ w505]
      tunnel: [i16 0 w504] -> w487
      tunnel: [T11."Enabled" ("禁用") T11."Disabled and Grayed Out" ("禁用")] -> w479
      tunnel: w476 -> [w499 _]
      frame False {
        n241 = case shown="真" w499 {
          frame False {
          }
          frame True {
            n242 = property on="柱塞泵3" class="Bool (严格)"("Val(Sgnl)"=FALSE ("值(信号)")) -> ()  [unwired: 2 in, 2 out]
          }
        }
      }
      frame True {
        n243 = Increment(x=w505) -> (x+1=w504:i16)
      }
    }
    n244 = case shown="假" w484 {
      tunnel: w489 -> [_ w512]
      tunnel: [i16 0 w511] -> w488
      tunnel: [T11."Enabled" ("禁用") T11."Disabled and Grayed Out" ("禁用")] -> w480
      tunnel: w477 -> [w506 _]
      frame False {
        n245 = case shown="真" w506 {
          frame False {
          }
          frame True {
            n246 = property on="柱塞泵2" class="Bool (严格)"("Val(Sgnl)"=FALSE ("值(信号)")) -> ()  [unwired: 2 in, 2 out]
          }
        }
      }
      frame True {
        n247 = Increment(x=w512) -> (x+1=w511:i16)
      }
    }
    n248 = property on="柱塞泵3" class="Bool (严格)"("DisabledEnum"=w479) -> ()  [unwired: 2 in, 2 out]
    n249 = property on="柱塞泵1" class="Bool (严格)"("DisabledEnum"=w495) -> ()  [unwired: 2 in, 2 out]
    n250 = property on="柱塞泵2" class="Bool (严格)"("DisabledEnum"=w480) -> ()  [unwired: 2 in, 2 out]
  }
  n251 = control-ref of="总磷加标水杯定容体积"() -> (w160:refnum<vi>)
  n252 = control-ref of="氨氮加标水杯定容体积"() -> (w202:refnum<vi>)
  n253 = Unbundle By Name(w195) -> ("量程"=→"氨氮量程":dbl, "检出限"=→"氨氮检出限":dbl, "加标前水样浓度"=→"氨氮加标前水样浓度":dbl, "加标后水样浓度"=→"氨氮加标后水样浓度":dbl, "加标水杯定容体积"=→"氨氮加标水杯定容体积":dbl, "加标母液浓度"=→"氨氮母液浓度":dbl, "加标体积"=→"氨氮加标体积":dbl, "加标回收率"=→"氨氮加标回收率":dbl)
  n254 = control-ref of="总磷加标前水样浓度"() -> (w162:refnum<vi>)
  n255 = control-ref of="总磷加标后水样浓度"() -> (w161:refnum<vi>)
  n256 = control-ref of="氨氮加标前水样浓度"() -> (w203:refnum<vi>)
  n257 = control-ref of="氨氮加标后水样浓度"() -> (w199:refnum<vi>)
  n258 = control-ref of="COD加标回收率"() -> (w148:refnum<vi>)
  n259 = control-ref of="COD母液浓度"() -> (w150:refnum<vi>)
  n260 = control-ref of="COD加标体积"() -> (w149:refnum<vi>)
  n261 = call "质控参数读取.vi"("section"="总磷质控参数", "error in (no error)"=w176) -> ("error out"=w173:errorcluster, "参数"=w185:T8)  [unwired: 8 in]
  n262 = control-ref of="总磷加标回收率"() -> (w158:refnum<vi>)
  n263 = control-ref of="氨氮加标回收率"() -> (w197:refnum<vi>)
  n264 = control-ref of="COD检出限"() -> (w154:refnum<vi>)
  n265 = control-ref of="总磷母液浓度"() -> (w159:refnum<vi>)
  n266 = control-ref of="总磷加标体积"() -> (w157:refnum<vi>)
  n267 = control-ref of="氨氮母液浓度"() -> (w201:refnum<vi>)
  n268 = control-ref of="氨氮加标体积"() -> (w198:refnum<vi>)
  n269 = control-ref of="COD量程"() -> (w155:refnum<vi>)
  n270 = control-ref of="总磷检出限"() -> (w163:refnum<vi>)
  n271 = control-ref of="氨氮检出限"() -> (w204:refnum<vi>)
  n272 = control-ref of="总磷量程"() -> (w164:refnum<vi>)
  n273 = control-ref of="氨氮量程"() -> (w205:refnum<vi>)
  n274 = Obtain Notifier(name (unnamed)="采配水Process" ("名称（未命名）"), notification data type=FALSE) -> (notifier out=w139:refnum<notifier>)  [unwired: 2 in, 2 out]
  n275 = Build Array(w155, w154, w153, w152, w151, w150, w149, w148) -> (w147:refnum<vi>[])
  n276 = Build Array(w164, w163, w162, w161, w160, w159, w157, w158) -> (w156:refnum<vi>[])
  n277 = Build Array(w205, w204, w203, w199, w202, w201, w198, w197) -> (w200:refnum<vi>[])
  n278 = Unbundle By Name(w185) -> ("量程"=→"总磷量程":dbl, "检出限"=→"总磷检出限":dbl, "加标前水样浓度"=→"总磷加标前水样浓度":dbl, "加标后水样浓度"=→"总磷加标后水样浓度":dbl, "加标水杯定容体积"=→"总磷加标水杯定容体积":dbl, "加标母液浓度"=→"总磷母液浓度":dbl, "加标体积"=→"总磷加标体积":dbl, "加标回收率"=→"总磷加标回收率":dbl)
  n279 = call "质控参数读取.vi"("section"="COD质控参数", "error in (no error)"=w173) -> ("error out"=w117:errorcluster, "参数"=w175:T8)  [unwired: 8 in]
  n280 = call "质控参数读取.vi"("section"="总氮质控参数", "error in (no error)"=w117) -> ("参数"=w116:T8)  [unwired: 8 in, 1 out]
  n281 = Unbundle By Name(w116) -> ("量程"=→"总氮量程":dbl, "检出限"=→"总氮检出限":dbl, "加标前水样浓度"=→"总氮加标前水样浓度":dbl, "加标后水样浓度"=→"总氮加标后水样浓度":dbl, "加标水杯定容体积"=→"总氮加标水杯定容体积":dbl, "加标母液浓度"=→"总氮母液浓度":dbl, "加标体积"=→"总氮加标体积":dbl, "加标回收率"=→"总氮加标回收率":dbl)
  n282 = Unbundle By Name(w175) -> ("量程"=→"COD量程":dbl, "检出限"=→"COD检出限":dbl, "加标前水样浓度"=→"COD加标前水样浓度":dbl, "加标后水样浓度"=→"COD加标后水样浓度":dbl, "加标水杯定容体积"=→"COD加标水杯定容体积":dbl, "加标母液浓度"=→"COD母液浓度":dbl, "加标体积"=→"COD加标体积":dbl, "加标回收率"=→"COD加标回收率":dbl)
  n283 = call <vilib>:"Application Directory.vi"() -> ("Application Directory"=w102:path)
  n284 = Build Path(base path=w102, name or relative path="data\\Set.ini" ("名称或相对路径")) -> (appended path=w100:path)
  n285 = call <vilib>:"Open Config Data.vi"("configuration file path"=w100) -> ("error out"=w98:errorcluster, "refnum"=w99:T13)  [unwired: 8 in, 1 out]
  n286 = call-poly <vilib>:"Read Key.vi"("section"=w96, "error in (no error)"=w98, "key"="背隙值1", "refnum"=w99) -> ("error out"=w93:errorcluster, "value"=w88:i32, "refnum out"=w95:T13)  [unwired: 4 in, 1 out]
  n287 = local write "背隙补偿步数"(w88) -> ()
  n288 = call-poly <vilib>:"Read Key.vi"("section"=w96, "error in (no error)"=w93, "key"="背隙值2", "refnum"=w95) -> ("error out"=w91:errorcluster, "value"=w89:i32, "refnum out"=w92:T13)  [unwired: 4 in, 1 out]
  n289 = Obtain Queue(name (unnamed)="采配水" ("名称（未命名）"), element data type=cluster{"命令":string, "数据":variant} {"命令"="", "数据"=variant}) -> (queue out=w129:refnum<queue>)  [unwired: 3 in, 2 out]
  n290 = while {
    tunnel: w200 -> [w525]
    tunnel: w156 -> [w524]
    tunnel: w147 -> [w523]
    tunnel: w139 -> [w522]
    tunnel: w129 -> [w521]
    tunnel: w119 -> [w520]
    stop <- FALSE stop-if-true
    # "氨氮站号是1，总磷总氮站号是2，COD站号是3"
    n291 = event shown="[42] \"氨氮加标回收启动\": 值改变" {
      selector: _ -> [_ _ _ _ _ _ _ _ _ _ _ _ _ _ _ _ _ _ _ _ _ _ _ _ _ _ _ _ _ _ _ _ _ _ _ _ _ _ _ _ _ _ _ _ _ _ _ _ _]
      dyn-events: _ -> [_ _ _ _ _ _ _ _ _ _ _ _ _ _ _ _ _ _ _ _ _ _ _ _ _ _ _ _ _ _ _ _ _ _ _ _ _ _ _ _ _ _ _ _ _ _ _ _ _]
      timeout: _ -> [_ _ _ _ _ _ _ _ _ _ _ _ _ _ _ _ _ _ _ _ _ _ _ _ _ _ _ _ _ _ _ _ _ _ _ _ _ _ _ _ _ _ _ _ _ _ _ _ _]
      tunnel: w525 -> [_ _ _ _ _ _ _ _ _ _ _ _ _ _ _ _ _ _ _ _ _ _ _ _ _ _ _ _ _ _ _ _ _ w849 _ _ _ w926 _ _ _ _ _ _ _ _ _ _ _]
      tunnel: w524 -> [_ _ _ _ _ _ _ _ _ _ _ _ _ _ _ _ _ _ _ _ _ _ _ _ _ _ _ _ _ _ _ _ _ _ w863 _ _ w923 _ _ _ _ _ _ _ _ _ _ _]
      tunnel: w523 -> [_ _ _ _ _ _ _ _ _ _ _ _ _ _ _ _ _ _ _ _ _ _ _ _ _ _ _ _ _ _ _ _ _ _ _ _ w901 w922 _ _ _ _ _ _ _ _ _ _ _]
      tunnel: w522 -> [_ _ _ _ _ _ _ _ _ _ _ _ _ _ _ _ _ _ _ _ _ _ _ _ _ _ _ _ _ _ _ _ _ _ _ _ _ _ _ _ w951 _ _ _ _ w1107 w1138 _ _]
      tunnel: w521 -> [_ _ _ _ _ _ _ _ _ _ _ _ _ _ _ _ _ _ _ _ _ _ _ _ _ _ _ _ _ _ _ _ _ _ _ _ _ _ _ _ _ _ _ _ _ _ w1135 _ _]
      tunnel: w520 -> [_ _ _ _ _ _ _ _ _ _ _ _ _ _ _ _ _ _ _ _ _ _ _ _ _ _ _ _ _ _ _ _ _ _ _ w881 _ w919 _ _ _ _ _ _ _ _ _ _ _]
      tunnel: [_ _ _ _ _ _ _ _ _ _ _ _ _ _ _ _ _ _ _ _ _ _ _ _ _ _ _ _ _ w785 w822 w829 w836 _ _ _ _ _ _ _ _ w982 _ _ _ _ _ _ _] -> _
      event Timeout {
        n292 = event-data() -> ()  [unwired: 1 in, 3 out]
      }
      event "氨氮量程", "氨氮检出限", "氨氮加标前水样浓度", "氨氮加标水杯定容体积", "氨氮母液浓度", "氨氮加标后水样浓度": Mouse Down {
        n293 = event-data() -> ("CtlRef"=w530:refnum<vi>)  [unwired: 1 in, 7 out]
        n294 = property class="DigNum (严格)"(reference=w530) -> (reference out=w528:refnum<vi>, "Value"=w529:dbl)  [unwired: 1 in, 1 out]
        n295 = call "数字键盘.vi"("OldNumber"=w529) -> ("NewNumber"=w527:sgl)
        n296 = property class="DigNum (严格)"(reference=w528, "Val(Sgnl)"=w527) -> ()  [unwired: 1 in, 2 out]
      }
      event "总磷母液浓度", "总磷加标水杯定容体积", "总磷加标后水样浓度", "总磷加标前水样浓度", "总磷检出限", "总磷量程": Mouse Down {
        n297 = event-data() -> ("CtlRef"=w534:refnum<vi>)  [unwired: 1 in, 7 out]
        n298 = property class="DigNum (严格)"(reference=w534) -> (reference out=w532:refnum<vi>, "Value"=w533:dbl)  [unwired: 1 in, 1 out]
        n299 = call "数字键盘.vi"("OldNumber"=w533) -> ("NewNumber"=w531:sgl)
        n300 = property class="DigNum (严格)"(reference=w532, "Val(Sgnl)"=w531) -> ()  [unwired: 1 in, 2 out]
      }
      event "总氮母液浓度", "总氮加标水杯定容体积", "总氮加标后水样浓度", "总氮加标前水样浓度", "总氮检出限", "总氮量程": Mouse Down {
        n301 = event-data() -> ("CtlRef"=w538:refnum<vi>)  [unwired: 1 in, 7 out]
        n302 = property class="DigNum (严格)"(reference=w538) -> (reference out=w536:refnum<vi>, "Value"=w537:dbl)  [unwired: 1 in, 1 out]
        n303 = call "数字键盘.vi"("OldNumber"=w537) -> ("NewNumber"=w535:sgl)
        n304 = property class="DigNum (严格)"(reference=w536, "Val(Sgnl)"=w535) -> ()  [unwired: 1 in, 2 out]
      }
      event "COD母液浓度", "COD加标水杯定容体积", "COD加标后水样浓度", "COD加标前水样浓度", "COD检出限", "COD量程": Mouse Down {
        n305 = event-data() -> ("CtlRef"=w542:refnum<vi>)  [unwired: 1 in, 7 out]
        n306 = property class="DigNum (严格)"(reference=w542) -> (reference out=w540:refnum<vi>, "Value"=w541:dbl)  [unwired: 1 in, 1 out]
        n307 = call "数字键盘.vi"("OldNumber"=w541) -> ("NewNumber"=w539:sgl)
        n308 = property class="DigNum (严格)"(reference=w540, "Val(Sgnl)"=w539) -> ()  [unwired: 1 in, 2 out]
      }
      event "背隙补偿步数": Mouse Down {
        n309 = event-data() -> ()  [unwired: 1 in, 8 out]
        n310 = local read "背隙补偿步数"() -> (w544:i32)
        n311 = call "数字键盘.vi"("OldNumber"=w544) -> ("NewNumber"=w543:sgl)
        n312 = local write "背隙补偿步数"(w543) -> ()
      }
      event "标准体积 1": Mouse Down {
        n313 = event-data() -> ()  [unwired: 1 in, 8 out]
        n314 = local read "标准体积 1"() -> (w546:dbl)
        n315 = call "数字键盘.vi"("OldNumber"=w546) -> ("NewNumber"=w545:sgl)
        n316 = local write "标准体积 1"(w545) -> ()
      }
      event "标准体积 2": Mouse Down {
        n317 = event-data() -> ()  [unwired: 1 in, 8 out]
        n318 = local read "标准体积 2"() -> (w548:dbl)
        n319 = call "数字键盘.vi"("OldNumber"=w548) -> ("NewNumber"=w547:sgl)
        n320 = local write "标准体积 2"(w547) -> ()
      }
      event "标准体积 3": Mouse Down {
        n321 = event-data() -> ()  [unwired: 1 in, 8 out]
        n322 = local read "标准体积 3"() -> (w550:dbl)
        n323 = call "数字键盘.vi"("OldNumber"=w550) -> ("NewNumber"=w549:sgl)
        n324 = local write "标准体积 3"(w549) -> ()
      }
      event "标准体积 4": Mouse Down {
        n325 = event-data() -> ()  [unwired: 1 in, 8 out]
        n326 = local read "标准体积 4"() -> (w552:dbl)
        n327 = call "数字键盘.vi"("OldNumber"=w552) -> ("NewNumber"=w551:sgl)
        n328 = local write "标准体积 4"(w551) -> ()
      }
      event "标准体积 5": Mouse Down {
        n329 = event-data() -> ()  [unwired: 1 in, 8 out]
        n330 = local read "标准体积 5"() -> (w554:dbl)
        n331 = call "数字键盘.vi"("OldNumber"=w554) -> ("NewNumber"=w553:sgl)
        n332 = local write "标准体积 5"(w553) -> ()
      }
      event "实际体积 1": Mouse Down {
        n333 = event-data() -> ()  [unwired: 1 in, 8 out]
        n334 = local read "实际体积 1"() -> (w556:dbl)
        n335 = call "数字键盘.vi"("OldNumber"=w556) -> ("NewNumber"=w555:sgl)
        n336 = local write "实际体积 1"(w555) -> ()
      }
      event "实际体积 2": Mouse Down {
        n337 = event-data() -> ()  [unwired: 1 in, 8 out]
        n338 = local read "实际体积 2"() -> (w558:dbl)
        n339 = call "数字键盘.vi"("OldNumber"=w558) -> ("NewNumber"=w557:sgl)
        n340 = local write "实际体积 2"(w557) -> ()
      }
      event "实际体积 3": Mouse Down {
        n341 = event-data() -> ()  [unwired: 1 in, 8 out]
        n342 = local read "实际体积 3"() -> (w560:dbl)
        n343 = call "数字键盘.vi"("OldNumber"=w560) -> ("NewNumber"=w559:sgl)
        n344 = local write "实际体积 3"(w559) -> ()
      }
      event "实际体积 4": Mouse Down {
        n345 = event-data() -> ()  [unwired: 1 in, 8 out]
        n346 = local read "实际体积 4"() -> (w562:dbl)
        n347 = call "数字键盘.vi"("OldNumber"=w562) -> ("NewNumber"=w561:sgl)
        n348 = local write "实际体积 4"(w561) -> ()
      }
      event "实际体积 5": Mouse Down {
        n349 = event-data() -> ()  [unwired: 1 in, 8 out]
        n350 = local read "实际体积 5"() -> (w564:dbl)
        n351 = call "数字键盘.vi"("OldNumber"=w564) -> ("NewNumber"=w563:sgl)
        n352 = local write "实际体积 5"(w563) -> ()
      }
      event "K": Mouse Down {
        n353 = event-data() -> ()  [unwired: 1 in, 8 out]
        n354 = local read "K"() -> (w566:dbl)
        n355 = call "数字键盘.vi"("OldNumber"=w566) -> ("NewNumber"=w565:sgl)
        n356 = local write "K"(w565) -> ()
      }
      event "B": Mouse Down {
        n357 = event-data() -> ()  [unwired: 1 in, 8 out]
        n358 = local read "B"() -> (w568:dbl)
        n359 = call "数字键盘.vi"("OldNumber"=w568) -> ("NewNumber"=w567:sgl)
        n360 = local write "B"(w567) -> ()
      }
      event "K 2": Mouse Down {
        n361 = event-data() -> ()  [unwired: 1 in, 8 out]
        n362 = local read "K 2"() -> (w570:dbl)
        n363 = call "数字键盘.vi"("OldNumber"=w570) -> ("NewNumber"=w569:sgl)
        n364 = local write "K 2"(w569) -> ()
      }
      event "B 2": Mouse Down {
        n365 = event-data() -> ()  [unwired: 1 in, 8 out]
        n366 = local read "B 2"() -> (w572:dbl)
        n367 = call "数字键盘.vi"("OldNumber"=w572) -> ("NewNumber"=w571:sgl)
        n368 = local write "B 2"(w571) -> ()
      }
      event "K 3": Mouse Down {
        n369 = event-data() -> ()  [unwired: 1 in, 8 out]
        n370 = local read "K 3"() -> (w574:dbl)
        n371 = call "数字键盘.vi"("OldNumber"=w574) -> ("NewNumber"=w573:sgl)
        n372 = local write "K 3"(w573) -> ()
      }
      event "B 3": Mouse Down {
        n373 = event-data() -> ()  [unwired: 1 in, 8 out]
        n374 = local read "B 3"() -> (w576:dbl)
        n375 = call "数字键盘.vi"("OldNumber"=w576) -> ("NewNumber"=w575:sgl)
        n376 = local write "B 3"(w575) -> ()
      }
      event "背隙补偿步数 2": Mouse Down {
        n377 = event-data() -> ()  [unwired: 1 in, 8 out]
        n378 = local read "背隙补偿步数 2"() -> (w577:i32)
        n379 = call "数字键盘.vi"("OldNumber"=w577) -> ("NewNumber"=w578:sgl)
        n380 = local write "背隙补偿步数 2"(w578) -> ()
      }
      event "背隙补偿步数 3": Mouse Down {
        n381 = event-data() -> ()  [unwired: 1 in, 8 out]
        n382 = local read "背隙补偿步数 3"() -> (w580:i32)
        n383 = call "数字键盘.vi"("OldNumber"=w580) -> ("NewNumber"=w579:sgl)
        n384 = local write "背隙补偿步数 3"(w579) -> ()
      }
      event "背隙补偿步数", "背隙补偿步数 2", "背隙补偿步数 3", "标准体积 1", "标准体积 2", "标准体积 3", "标准体积 4", "标准体积 5", "实际体积 1", "实际体积 2", "实际体积 3", "实际体积 4", "实际体积 5": Value Change {
        w601 = "质控线性参数" ("section")
        w632 = "质控背隙补偿" ("section")
        n385 = event-data() -> ()  [unwired: 1 in, 6 out]
        n386 = call <vilib>:"Application Directory.vi"() -> ("Application Directory"=w639:path)
        n387 = Build Path(base path=w639, name or relative path="data\\Set.ini" ("名称或相对路径")) -> (appended path=w637:path)
        n388 = call <vilib>:"Open Config Data.vi"("configuration file path"=w637) -> ("error out"=w635:errorcluster, "refnum"=w636:T13)  [unwired: 8 in, 1 out]
        n389 = call-poly <vilib>:"Write Key.vi"("section"=w632, "error in (no error)"=w635, "value"="背隙补偿步数", "key"="背隙值1", "refnum"=w636) -> ("error out"=w626:errorcluster, "refnum out"=w629:T13)  [unwired: 4 in, 1 out]
        n390 = call-poly <vilib>:"Write Key.vi"("section"=w632, "error in (no error)"=w626, "value"="背隙补偿步数 2", "key"="背隙值2", "refnum"=w629) -> ("error out"=w627:errorcluster, "refnum out"=w628:T13)  [unwired: 4 in, 1 out]
        n391 = local read "标准体积 1"() -> (w599:dbl)
        n392 = call-poly <vilib>:"Write Key.vi"("section"=w632, "error in (no error)"=w627, "value"="背隙补偿步数 3", "key"="背隙值3", "refnum"=w628) -> ("error out"=w622:errorcluster, "refnum out"=w623:T13)  [unwired: 4 in, 1 out]
        n393 = local read "标准体积 2"() -> (w598:dbl)
        n394 = local read "标准体积 3"() -> (w596:dbl)
        n395 = call-poly <vilib>:"Write Key.vi"("section"=w601, "error in (no error)"=w622, "value"=w599, "key"="标准体积1", "refnum"=w623) -> ("error out"=w620:errorcluster, "refnum out"=w621:T13)  [unwired: 4 in, 1 out]
        n396 = local read "标准体积 4"() -> (w592:dbl)
        n397 = call-poly <vilib>:"Write Key.vi"("section"=w601, "error in (no error)"=w620, "value"=w598, "key"="标准体积2", "refnum"=w621) -> ("error out"=w618:errorcluster, "refnum out"=w619:T13)  [unwired: 4 in, 1 out]
        n398 = call-poly <vilib>:"Write Key.vi"("section"=w601, "error in (no error)"=w618, "value"=w596, "key"="标准体积3", "refnum"=w619) -> ("error out"=w616:errorcluster, "refnum out"=w617:T13)  [unwired: 4 in, 1 out]
        n399 = local read "标准体积 5"() -> (w591:dbl)
        n400 = call-poly <vilib>:"Write Key.vi"("section"=w601, "error in (no error)"=w616, "value"=w592, "key"="标准体积4", "refnum"=w617) -> ("error out"=w614:errorcluster, "refnum out"=w615:T13)  [unwired: 4 in, 1 out]
        n401 = local read "实际体积 1"() -> (w585:dbl)
        n402 = call-poly <vilib>:"Write Key.vi"("section"=w601, "error in (no error)"=w614, "value"=w591, "key"="标准体积5", "refnum"=w615) -> ("error out"=w612:errorcluster, "refnum out"=w613:T13)  [unwired: 4 in, 1 out]
        n403 = local read "实际体积 2"() -> (w584:dbl)
        n404 = call-poly <vilib>:"Write Key.vi"("section"=w601, "error in (no error)"=w612, "value"=w585, "key"="实际体积1", "refnum"=w613) -> ("error out"=w610:errorcluster, "refnum out"=w611:T13)  [unwired: 4 in, 1 out]
        n405 = local read "实际体积 3"() -> (w583:dbl)
        n406 = local read "实际体积 4"() -> (w582:dbl)
        n407 = call-poly <vilib>:"Write Key.vi"("section"=w601, "error in (no error)"=w610, "value"=w584, "key"="实际体积2", "refnum"=w611) -> ("error out"=w608:errorcluster, "refnum out"=w609:T13)  [unwired: 4 in, 1 out]
        n408 = local read "实际体积 5"() -> (w581:dbl)
        n409 = call-poly <vilib>:"Write Key.vi"("section"=w601, "error in (no error)"=w608, "value"=w583, "key"="实际体积3", "refnum"=w609) -> ("error out"=w606:errorcluster, "refnum out"=w607:T13)  [unwired: 4 in, 1 out]
        n410 = call-poly <vilib>:"Write Key.vi"("section"=w601, "error in (no error)"=w606, "value"=w582, "key"="实际体积4", "refnum"=w607) -> ("error out"=w604:errorcluster, "refnum out"=w605:T13)  [unwired: 4 in, 1 out]
        n411 = call-poly <vilib>:"Write Key.vi"("section"=w601, "error in (no error)"=w604, "value"=w581, "key"="实际体积5", "refnum"=w605) -> ("error out"=w602:errorcluster, "refnum out"=w603:T13)  [unwired: 4 in, 1 out]
        n412 = call <vilib>:"Close Config Data.vi"("error in (no error)"=w602, "refnum"=w603) -> ()  [unwired: 8 in, 2 out]
      }
      event "氨氮", "总磷总氮", "CODMn", "总磷模块选择": Value Change {
        w642 = "质控模块选择" ("section")
        n413 = event-data() -> ()  [unwired: 1 in, 6 out]
        n414 = call <vilib>:"Application Directory.vi"() -> ("Application Directory"=w661:path)
        n415 = Build Path(base path=w661, name or relative path="data\\Set.ini" ("名称或相对路径")) -> (appended path=w659:path)
        n416 = call <vilib>:"Open Config Data.vi"("configuration file path"=w659) -> ("error out"=w657:errorcluster, "refnum"=w658:T13)  [unwired: 8 in, 1 out]
        n417 = local read "氨氮"() -> (w649:bool)
        n418 = local read "总磷总氮"() -> (w648:bool)
        n419 = call-poly <vilib>:"Write Key.vi"("section"=w642, "error in (no error)"=w657, "value"=w649, "key"="模块1" ("section"), "refnum"=w658) -> ("error out"=w655:errorcluster, "refnum out"=w656:T13)  [unwired: 4 in, 1 out]
        n420 = local read "CODMn"() -> (w647:bool)
        n421 = call-poly <vilib>:"Write Key.vi"("section"=w642, "error in (no error)"=w655, "value"=w648, "key"="模块2" ("section"), "refnum"=w656) -> ("error out"=w653:errorcluster, "refnum out"=w654:T13)  [unwired: 4 in, 1 out]
        n422 = call-poly <vilib>:"Write Key.vi"("section"=w642, "error in (no error)"=w653, "value"=w647, "key"="模块3" ("section"), "refnum"=w654) -> ("error out"=w645:errorcluster, "refnum out"=w646:T13)  [unwired: 4 in, 1 out]
        n423 = local read "总磷模块选择"() -> (w640:enum32{"氨氮总磷", "总氮总磷"})
        n424 = call-poly <vilib>:"Write Key.vi"("section"=w642, "error in (no error)"=w645, "value"=w640, "key"="总磷模块" ("section"), "refnum"=w646) -> ("error out"=w643:errorcluster, "refnum out"=w644:T13)  [unwired: 4 in, 1 out]
        n425 = call <vilib>:"Close Config Data.vi"("error in (no error)"=w643, "refnum"=w644) -> ()  [unwired: 8 in, 2 out]
      }
      event "氨氮量程选择", "总氮量程选择", "总磷量程选择", "CODMn量程选择": Value Change {
        w666 = "质控模块量程选择" ("section")
        n426 = event-data() -> ()  [unwired: 1 in, 6 out]
        n427 = call <vilib>:"Application Directory.vi"() -> ("Application Directory"=w683:path)
        n428 = Build Path(base path=w683, name or relative path="data\\Set.ini" ("名称或相对路径")) -> (appended path=w681:path)
        n429 = local read "氨氮量程选择"() -> (w665:enum32{"H", "L", "AUTO"})
        n430 = call <vilib>:"Open Config Data.vi"("configuration file path"=w681) -> ("error out"=w679:errorcluster, "refnum"=w680:T13)  [unwired: 8 in, 1 out]
        n431 = local read "总氮量程选择"() -> (w664:enum32{"H", "L", "AUTO"})
        n432 = call-poly <vilib>:"Write Key.vi"("section"=w666, "error in (no error)"=w679, "value"=w665, "key"="氨氮" ("section"), "refnum"=w680) -> ("error out"=w677:errorcluster, "refnum out"=w678:T13)  [unwired: 4 in, 1 out]
        n433 = local read "总磷量程选择"() -> (w663:enum32{"H", "L", "AUTO"})
        n434 = call-poly <vilib>:"Write Key.vi"("section"=w666, "error in (no error)"=w677, "value"=w664, "key"="总氮" ("section"), "refnum"=w678) -> ("error out"=w675:errorcluster, "refnum out"=w676:T13)  [unwired: 4 in, 1 out]
        n435 = local read "CODMn量程选择"() -> (w662:enum32{"H", "L", "AUTO"})
        n436 = call-poly <vilib>:"Write Key.vi"("section"=w666, "error in (no error)"=w675, "value"=w663, "key"="总磷" ("section"), "refnum"=w676) -> ("error out"=w670:errorcluster, "refnum out"=w671:T13)  [unwired: 4 in, 1 out]
        n437 = call-poly <vilib>:"Write Key.vi"("section"=w666, "error in (no error)"=w670, "value"=w662, "key"="CODMn" ("section"), "refnum"=w671) -> ("error out"=w668:errorcluster, "refnum out"=w669:T13)  [unwired: 4 in, 1 out]
        n438 = call <vilib>:"Close Config Data.vi"("error in (no error)"=w668, "refnum"=w669) -> ()  [unwired: 8 in, 2 out]
      }
      event "写入": Value Change {
        n439 = event-data() -> ()  [unwired: 1 in, 6 out]
        n440 = local read "枚举"() -> (w685:enum16{"柱塞泵1", "柱塞泵2", "柱塞泵3"})
        n441 = case shown="\"柱塞泵3\"" w685 {
          tunnel: [w686 w698 w709] -> w684
          frame "柱塞泵1", Default {
            n442 = local read "K"() -> (w690:dbl)
            n443 = local read "B"() -> (w691:dbl)
            n444 = local read "背隙补偿步数"() -> (w687:i32)
            n445 = Build Array(w690, w691) -> (w692:dbl[])
            n446 = call "浮点转CDAB整形ZK.vi"("浮点数"=w692) -> ("CDAB整形输出"=w694:u16[])  [unwired: 10 in]
            n447 = Build Array(w687) -> (w693:i32[])
            n448 = Insert Into Array(array=w693, index=0 ("索引"), new element=w694) -> (w696:i32[])
            n449 = call "写入参数.vi"("values"=w696, "starting address"=u16 1, "Slave ID"=u8 1) -> ("error out"=w686:errorcluster)  [unwired: 8 in]
          }
          frame "柱塞泵2" {
            n450 = local read "背隙补偿步数 2"() -> (w700:i32)
            n451 = local read "K 2"() -> (w703:dbl)
            n452 = local read "B 2"() -> (w702:dbl)
            n453 = Build Array(w703, w702) -> (w704:dbl[])
            n454 = call "浮点转CDAB整形ZK.vi"("浮点数"=w704) -> ("CDAB整形输出"=w705:u16[])  [unwired: 10 in]
            n455 = Build Array(w700) -> (w699:i32[])
            n456 = Insert Into Array(array=w699, index=0 ("索引"), new element=w705) -> (w707:i32[])
            n457 = call "写入参数.vi"("values"=w707, "starting address"=u16 1, "Slave ID"=u8 2) -> ("error out"=w698:errorcluster)  [unwired: 8 in]
          }
          frame "柱塞泵3" {
            n458 = local read "背隙补偿步数 3"() -> (w711:i32)
            n459 = local read "K 3"() -> (w715:dbl)
            n460 = local read "B 3"() -> (w716:dbl)
            n461 = Build Array(w715, w716) -> (w717:dbl[])
            n462 = call "浮点转CDAB整形ZK.vi"("浮点数"=w717) -> ("CDAB整形输出"=w718:u16[])  [unwired: 10 in]
            n463 = Build Array(w711) -> (w713:i32[])
            n464 = Insert Into Array(array=w713, index=0 ("索引"), new element=w718) -> (w712:i32[])
            n465 = call "写入参数.vi"("values"=w712, "starting address"=u16 1, "Slave ID"=u8 3) -> ("error out"=w709:errorcluster)  [unwired: 8 in]
          }
        }
        n466 = case shown="无错误" w684 {
          frame No Error {
            n467 = One Button Dialog(message="写入成功" ("消息"), button name ("OK")="确定" ("按钮名称（“确定”）")) -> ()  [unwired: 1 out]
          }
          frame Error {
            n468 = One Button Dialog(message="写入失败" ("消息"), button name ("OK")="确定" ("按钮名称（“确定”）")) -> ()  [unwired: 1 out]
          }
        }
      }
      event "读取": Value Change {
        n469 = event-data() -> ()  [unwired: 1 in, 6 out]
        n470 = local read "氨氮"() -> (w723:bool)
        n471 = case shown="假" w723 {
          tunnel: [errorcluster {"status"=FALSE, "code"=0, "source"=""} ("error out") w745] -> w736
          tunnel: [w738 w742] -> w733
          tunnel: [w737 w741] -> w732
          frame False {
            n472 = local read "簇"() -> (w739:T1)
            n473 = Unbundle By Name(w739) -> ("K3"=w738:sgl, "B3"=w737:sgl)
          }
          frame True {
            n474 = call "读取参数.vi"("Slave ID"=u8 1, "starting address"=u16 1, "quantity"=u16 4) -> ("values"=w744:u16[], "error out"=w745:errorcluster)  [unwired: 6 in]
            n475 = call "浮点CDAB转换质控.vi"("数组"=w744) -> ("数组 2"=w743:sgl[])  [unwired: 10 in]
            n476 = Index Array(array=w743) -> (element #1=w742:sgl, element #2=w741:sgl)  [unwired: 2 in]
          }
        }
        n477 = local read "总磷总氮"() -> (w724:bool)
        n478 = case shown="假" w724 {
          tunnel: w736 -> [w749 w760]
          tunnel: [w749 w759] -> w735
          tunnel: [w751 w756] -> w731
          tunnel: [w750 w755] -> w730
          frame False {
            n479 = local read "簇"() -> (w752:T1)
            n480 = Unbundle By Name(w752) -> ("K3"=w751:sgl, "B3"=w750:sgl)
          }
          frame True {
            n481 = call "读取参数.vi"("Slave ID"=u8 2, "starting address"=u16 1, "quantity"=u16 4, "Error in"=w760) -> ("values"=w758:u16[], "error out"=w759:errorcluster)  [unwired: 5 in]
            n482 = call "浮点CDAB转换质控.vi"("数组"=w758) -> ("数组 2"=w757:sgl[])  [unwired: 10 in]
            n483 = Index Array(array=w757) -> (element #1=w756:sgl, element #2=w755:sgl)  [unwired: 2 in]
          }
        }
        n484 = local read "CODMn"() -> (w725:bool)
        n485 = case shown="假" w725 {
          tunnel: w735 -> [w762 w773]
          tunnel: [w764 w770] -> w729
          tunnel: [w763 w769] -> w728
          tunnel: [w762 w766] -> w726
          frame False {
            n486 = local read "簇"() -> (w765:T1)
            n487 = Unbundle By Name(w765) -> ("K3"=w764:sgl, "B3"=w763:sgl)
          }
          frame True {
            n488 = call "读取参数.vi"("Slave ID"=u8 3, "starting address"=u16 1, "quantity"=u16 4, "Error in"=w773) -> ("values"=w772:u16[], "error out"=w766:errorcluster)  [unwired: 5 in]
            n489 = call "浮点CDAB转换质控.vi"("数组"=w772) -> ("数组 2"=w771:sgl[])  [unwired: 10 in]
            n490 = Index Array(array=w771) -> (element #1=w770:sgl, element #2=w769:sgl)  [unwired: 2 in]
          }
        }
        n491 = Bundle By Name(cluster=T1 {"K1"=0.0, "B1"=0.0, "K2"=0.0, "B2"=0.0, "K3"=0.0, "B3"=0.0} ("簇"), "K1"=w733, "B1"=w732, "K2"=w731, "B2"=w730, "K3"=w729, "B3"=w728) -> (→"簇":T1)
        n492 = case shown="无错误" w726 {
          frame No Error {
            n493 = One Button Dialog(message="读取成功" ("消息"), button name ("OK")="确定" ("按钮名称（“确定”）")) -> ()  [unwired: 1 out]
          }
          frame Error {
            n494 = One Button Dialog(message="读取失败" ("消息"), button name ("OK")="确定" ("按钮名称（“确定”）")) -> ()  [unwired: 1 out]
          }
        }
      }
      event "注出体积选择": Value Change {
        n495 = event-data() -> ()  [unwired: 1 in, 6 out]
        n496 = case shown="0" "注出体积选择" {
          tunnel: [0.1 0.3 0.5 0.8 1.0] -> w796
          frame 0 {
          }
          frame 1 {
          }
          frame 2 {
          }
          frame 3 {
          }
          frame 4, Default {
          }
        }
        n497 = local read "氨氮"() -> (w781:bool)
        n498 = Build Array(w796) -> (w783:dbl[])
        n499 = call "浮点转CDAB整形ZK.vi"("浮点数"=w783) -> ("CDAB整形输出"=w782:u16[])  [unwired: 10 in]
        n500 = case shown="假" w781 {
          tunnel: [_ w803] -> w799
          tunnel: [u16 8 ("starting address") w802] -> w797
          tunnel: w782 -> [_ w801]
          frame False {
          }
          frame True {
            w802 = u16 8 ("starting address")
            n501 = call "写入参数.vi"("values"=w801, "starting address"=w802, "Slave ID"=u8 1) -> ("error out"=w803:errorcluster)  [unwired: 8 in]
          }
        }
        n502 = local read "总磷总氮"() -> (w780:bool)
        n503 = case shown="真" w780 {
          tunnel: w799 -> [w805 w809]
          tunnel: [w805 w808] -> w798
          tunnel: w797 -> [_ w807]
          tunnel: w782 -> [_ w806]
          frame False {
          }
          frame True {
            n504 = call "写入参数.vi"("Error in"=w809, "values"=w806, "starting address"=w807, "Slave ID"=u8 2) -> ("error out"=w808:errorcluster)  [unwired: 7 in]
          }
        }
        n505 = local read "CODMn"() -> (w779:bool)
        n506 = case shown="真" w779 {
          tunnel: w798 -> [w811 w815]
          tunnel: w797 -> [_ w814]
          tunnel: [w811 w813] -> w792
          tunnel: w782 -> [_ w812]
          frame False {
          }
          frame True {
            n507 = call "写入参数.vi"("Error in"=w815, "values"=w812, "starting address"=w814, "Slave ID"=u8 3) -> ("error out"=w813:errorcluster)  [unwired: 7 in]
          }
        }
        n508 = call <vilib>:"Application Directory.vi"() -> ("Application Directory"=w795:path)
        n509 = Build Path(base path=w795, name or relative path="data\\Set.ini" ("名称或相对路径")) -> (appended path=w793:path)
        n510 = call <vilib>:"Open Config Data.vi"("error in (no error)"=w792, "configuration file path"=w793) -> ("error out"=w788:errorcluster, "refnum"=w789:T13)  [unwired: 7 in, 1 out]
        n511 = call-poly <vilib>:"Write Key.vi"("section"="质控手动体积选择", "error in (no error)"=w788, "value"="注出体积选择", "key"="手动体积选择" ("section"), "refnum"=w789) -> ("error out"=w790:errorcluster, "refnum out"=w791:T13)  [unwired: 4 in, 1 out]
        n512 = call <vilib>:"Close Config Data.vi"("error in (no error)"=w790, "refnum"=w791) -> ("error out"=w785:errorcluster)  [unwired: 8 in, 1 out]
      }
      event "柱塞泵1": Value Change {
        n513 = event-data() -> ()  [unwired: 1 in, 6 out]
        n514 = Build Array("柱塞泵1") -> (w823:bool[])
        n515 = call "多个线圈写入.vi"("values"=w823, "starting address"=u16 2104, "Slave ID"=u8 1) -> ("error out"=w822:errorcluster)  [unwired: 8 in]
        n516 = case shown="错误" w822 {
          frame No Error {
          }
          frame Error {
            n517 = One Button Dialog(message="启动失败" ("消息"), button name ("OK")="确定" ("按钮名称（“确定”）")) -> ()  [unwired: 1 out]
          }
        }
      }
      event "柱塞泵2": Value Change {
        n518 = event-data() -> ()  [unwired: 1 in, 6 out]
        n519 = Build Array("柱塞泵2") -> (w831:bool[])
        n520 = call "多个线圈写入.vi"("values"=w831, "starting address"=u16 2104, "Slave ID"=u8 2) -> ("error out"=w829:errorcluster)  [unwired: 8 in]
        n521 = case shown="错误" w829 {
          frame No Error {
          }
          frame Error {
            n522 = One Button Dialog(message="启动失败" ("消息"), button name ("OK")="确定" ("按钮名称（“确定”）")) -> ()  [unwired: 1 out]
          }
        }
      }
      event "柱塞泵3": Value Change {
        n523 = event-data() -> ()  [unwired: 1 in, 6 out]
        n524 = Build Array("柱塞泵3") -> (w838:bool[])
        n525 = call "多个线圈写入.vi"("values"=w838, "starting address"=u16 2104, "Slave ID"=u8 3) -> ("error out"=w836:errorcluster)  [unwired: 8 in]
        n526 = case shown="无错误" w836 {
          frame No Error {
          }
          frame Error {
            n527 = One Button Dialog(message="启动失败" ("消息"), button name ("OK")="确定" ("按钮名称（“确定”）")) -> ()  [unwired: 1 out]
          }
        }
      }
      event "氨氮量程", "氨氮检出限", "氨氮加标前水样浓度", "氨氮母液浓度", "氨氮加标水杯定容体积", "氨氮加标后水样浓度": Value Change {
        n528 = event-data() -> ()  [unwired: 1 in, 6 out]
        n529 = for {
          tunnel: w849 -> [w861] mode=indexing
          tunnel: [w860] -> w858 mode=indexing
          n530 = property class="DigNum (严格)"(reference=w861) -> ("Value"=w860:dbl)  [unwired: 1 in, 2 out]
        }
        n531 = Index Array(array=w858) -> (element #1=w857:dbl, element #2=w856:dbl, element #3=w843:dbl, element #4=w855:dbl, element #5=w854:dbl, element #6=w852:dbl)  [unwired: 6 in]
        n532 = Bundle By Name(cluster=T8 {"量程"=0.0, "检出限"=0.0, "加标前水样浓度"=0.0, "加标后水样浓度"=0.0, "加标水杯定容体积"=0.0, "加标母液浓度"=0.0, "加标体积"=0.0, "加标回收率"=0.0} ("参数"), "量程"=w857, "检出限"=w856, "加标前水样浓度"=w843, "加标后水样浓度"=w855, "加标水杯定容体积"=w854, "加标母液浓度"=w852) -> (w851:T8)
        n533 = global write "水样浓度全局.vi" "氨氮加标前水样浓度"(w843) -> ()
        n534 = call "加标回收率计算.vi"("参数"=w851) -> ("参数 out"=w850:T8)  [unwired: 10 in]
        n535 = Index Array(array=w849, index #1=6 ("索引")) -> (element #1=w848:refnum<vi>, element #2=w846:refnum<vi>)  [unwired: 1 in]
        n536 = call "质控参数保存.vi"("section"="氨氮质控参数", "参数"=w850) -> ()  [unwired: 9 in, 1 out]
        n537 = Unbundle By Name(w850) -> ("加标体积"=w844:dbl, "加标回收率"=w845:dbl)
        n538 = property class="DigNum (严格)"(reference=w848, "Value"=w844) -> ()  [unwired: 1 in, 2 out]
        n539 = property class="DigNum (严格)"(reference=w846, "Value"=w845) -> ()  [unwired: 1 in, 2 out]
      }
      event "总磷母液浓度", "总磷加标水杯定容体积", "总磷加标后水样浓度", "总磷加标前水样浓度", "总磷检出限", "总磷量程": Value Change {
        n540 = event-data() -> ()  [unwired: 1 in, 6 out]
        n541 = for {
          tunnel: w863 -> [w880] mode=indexing
          tunnel: [w879] -> w877 mode=indexing
          n542 = property class="DigNum (严格)"(reference=w880) -> ("Value"=w879:dbl)  [unwired: 1 in, 2 out]
        }
        n543 = Index Array(array=w877) -> (element #1=w876:dbl, element #2=w875:dbl, element #3=w862:dbl, element #4=w874:dbl, element #5=w873:dbl, element #6=w871:dbl)  [unwired: 6 in]
        n544 = global write "水样浓度全局.vi" "总磷加标前水样浓度"(w862) -> ()
        n545 = Bundle By Name(cluster=T8 {"量程"=0.0, "检出限"=0.0, "加标前水样浓度"=0.0, "加标后水样浓度"=0.0, "加标水杯定容体积"=0.0, "加标母液浓度"=0.0, "加标体积"=0.0, "加标回收率"=0.0} ("参数"), "量程"=w876, "检出限"=w875, "加标前水样浓度"=w862, "加标后水样浓度"=w874, "加标水杯定容体积"=w873, "加标母液浓度"=w871) -> (w870:T8)
        n546 = call "加标回收率计算.vi"("参数"=w870) -> ("参数 out"=w869:T8)  [unwired: 10 in]
        n547 = Index Array(array=w863, index #1=6 ("索引")) -> (element #1=w868:refnum<vi>, element #2=w865:refnum<vi>)  [unwired: 1 in]
        n548 = call "质控参数保存.vi"("section"="总磷质控参数", "参数"=w869) -> ()  [unwired: 9 in, 1 out]
        n549 = Unbundle By Name(w869) -> ("加标体积"=w866:dbl, "加标回收率"=w864:dbl)
        n550 = property class="DigNum (严格)"(reference=w868, "Value"=w866) -> ()  [unwired: 1 in, 2 out]
        n551 = property class="DigNum (严格)"(reference=w865, "Value"=w864) -> ()  [unwired: 1 in, 2 out]
      }
      event "总氮量程", "总氮检出限", "总氮加标前水样浓度", "总氮加标后水样浓度", "总氮加标水杯定容体积", "总氮母液浓度": Value Change {
        n552 = event-data() -> ()  [unwired: 1 in, 6 out]
        n553 = for {
          tunnel: w881 -> [w899] mode=indexing
          tunnel: [w898] -> w896 mode=indexing
          n554 = property class="DigNum (严格)"(reference=w899) -> ("Value"=w898:dbl)  [unwired: 1 in, 2 out]
        }
        n555 = Index Array(array=w896) -> (element #1=w895:dbl, element #2=w894:dbl, element #3=w882:dbl, element #4=w893:dbl, element #5=w892:dbl, element #6=w890:dbl)  [unwired: 6 in]
        n556 = global write "水样浓度全局.vi" "总氮加标前水样浓度"(w882) -> ()
        n557 = Bundle By Name(cluster=T8 {"量程"=0.0, "检出限"=0.0, "加标前水样浓度"=0.0, "加标后水样浓度"=0.0, "加标水杯定容体积"=0.0, "加标母液浓度"=0.0, "加标体积"=0.0, "加标回收率"=0.0} ("参数"), "量程"=w895, "检出限"=w894, "加标前水样浓度"=w882, "加标后水样浓度"=w893, "加标水杯定容体积"=w892, "加标母液浓度"=w890) -> (w889:T8)
        n558 = call "加标回收率计算.vi"("参数"=w889) -> ("参数 out"=w888:T8)  [unwired: 10 in]
        n559 = Index Array(array=w881, index #1=6 ("索引")) -> (element #1=w887:refnum<vi>, element #2=w884:refnum<vi>)  [unwired: 1 in]
        n560 = call "质控参数保存.vi"("section"="总氮质控参数", "参数"=w888) -> ()  [unwired: 9 in, 1 out]
        n561 = Unbundle By Name(w888) -> ("加标体积"=w885:dbl, "加标回收率"=w883:dbl)
        n562 = property class="DigNum (严格)"(reference=w887, "Value"=w885) -> ()  [unwired: 1 in, 2 out]
        n563 = property class="DigNum (严格)"(reference=w884, "Value"=w883) -> ()  [unwired: 1 in, 2 out]
      }
      event "COD母液浓度", "COD加标水杯定容体积", "COD加标后水样浓度", "COD加标前水样浓度", "COD检出限", "COD量程": Value Change {
        n564 = event-data() -> ()  [unwired: 1 in, 6 out]
        n565 = for {
          tunnel: w901 -> [w918] mode=indexing
          tunnel: [w917] -> w915 mode=indexing
          n566 = property class="DigNum (严格)"(reference=w918) -> ("Value"=w917:dbl)  [unwired: 1 in, 2 out]
        }
        n567 = Index Array(array=w915) -> (element #1=w914:dbl, element #2=w913:dbl, element #3=w900:dbl, element #4=w912:dbl, element #5=w911:dbl, element #6=w909:dbl)  [unwired: 6 in]
        n568 = global write "水样浓度全局.vi" "COD加标前水样浓度"(w900) -> ()
        n569 = Bundle By Name(cluster=T8 {"量程"=0.0, "检出限"=0.0, "加标前水样浓度"=0.0, "加标后水样浓度"=0.0, "加标水杯定容体积"=0.0, "加标母液浓度"=0.0, "加标体积"=0.0, "加标回收率"=0.0} ("参数"), "量程"=w914, "检出限"=w913, "加标前水样浓度"=w900, "加标后水样浓度"=w912, "加标水杯定容体积"=w911, "加标母液浓度"=w909) -> (w908:T8)
        n570 = call "加标回收率计算.vi"("参数"=w908) -> ("参数 out"=w907:T8)  [unwired: 10 in]
        n571 = Index Array(array=w901, index #1=6 ("索引")) -> (element #1=w906:refnum<vi>, element #2=w903:refnum<vi>)  [unwired: 1 in]
        n572 = call "质控参数保存.vi"("section"="COD质控参数", "参数"=w907) -> ()  [unwired: 9 in, 1 out]
        n573 = Unbundle By Name(w907) -> ("加标体积"=w904:dbl, "加标回收率"=w902:dbl)
        n574 = property class="DigNum (严格)"(reference=w906, "Value"=w904) -> ()  [unwired: 1 in, 2 out]
        n575 = property class="DigNum (严格)"(reference=w903, "Value"=w902) -> ()  [unwired: 1 in, 2 out]
      }
      event "氨氮调试", "总磷调试", "CODMn调试", "总氮调试": Value Change {
        n576 = event-data() -> ("CtlRef"=w925:refnum<vi>)  [unwired: 1 in, 5 out]
        n577 = property class="Bool"(reference=w925) -> ("Label.Text"=w924:string)  [unwired: 1 in, 2 out]
        n578 = case shown="\"CODMn调试\"" w924 {
          tunnel: w926 -> [w927 _ _ _]
          tunnel: w923 -> [_ w929 _ _]
          tunnel: w922 -> [_ _ _ w933]
          tunnel: ["氨氮模块" ("标题") "总磷模块" ("标题") "总氮模块" ("标题") "CODMn模块" ("标题")] -> w921
          tunnel: [w927 w929 w931 w933] -> w920
          tunnel: w919 -> [_ _ w931 _]
          frame "氨氮调试", Default {
          }
          frame "总磷调试" {
          }
          frame "总氮调试" {
          }
          frame "CODMn调试" {
          }
        }
        n579 = call "加标模块单控对话框.vi"("数组"=w920, "标题"=w921) -> ()  [unwired: 10 in]
      }
      event "氨氮停止", "总磷停止", "CODMn停止", "总氮停止": Value Change {
        n580 = event-data() -> ("CtlRef"=w939:refnum<vi>)  [unwired: 1 in, 5 out]
        n581 = property class="Bool"(reference=w939) -> ("Label.Text"=w938:string)  [unwired: 1 in, 2 out]
        n582 = case shown="\"总氮停止\", \"总磷停止\"" w938 {
          tunnel: [u8 1 ("Slave ID") u8 2 ("Slave ID") u8 3 ("Slave ID")] -> w935
          frame "氨氮停止", Default {
          }
          frame "总氮停止", "总磷停止" {
          }
          frame "CODMn停止" {
          }
        }
        n583 = call "单个写入.vi"("value"=u16 2, "address"=u16 103, "Slave ID"=w935) -> ()  [unwired: 8 in, 1 out]
      }
      event "氨氮排液", "CODMn排液", "总磷排液", "总氮排液": Value Change {
        n584 = event-data() -> ("CtlRef"=w947:refnum<vi>)  [unwired: 1 in, 5 out]
        n585 = property class="Bool"(reference=w947) -> ("Label.Text"=w946:string)  [unwired: 1 in, 2 out]
        n586 = case shown="\"CODMn排液\"" w946 {
          tunnel: [u8 1 ("Slave ID") u8 2 ("Slave ID") u8 3 ("Slave ID")] -> w943
          frame "氨氮排液", Default {
          }
          frame "总氮排液", "总磷排液" {
          }
          frame "CODMn排液" {
          }
        }
        n587 = call "单个写入.vi"("value"=u16 3, "address"=u16 103, "Slave ID"=w943) -> ()  [unwired: 8 in, 1 out]
      }
      event "加标回收": Value Change {
        n588 = event-data() -> ()  [unwired: 1 in, 6 out]
        n589 = flat-sequence {
          tunnel: [w955] -> w954
          tunnel: [w959] -> w953
          tunnel: [w958] -> w952
          tunnel: w951 -> [w956]
          tunnel: w954 -> [w967]
          tunnel: w953 -> [w966]
          tunnel: w952 -> [w965]
          frame #0 {
            n590 = Send Notification(notification=FALSE ("通知"), notifier=w956) -> ()  [unwired: 1 in, 2 out]
            n591 = call "质控启动流程对话框.vi"() -> ("启动模块"=w955:T3, "直接启动"=w958:bool, "常规启动"=w959:bool)  [unwired: 8 in, 1 out]
            "常规启动" <- w959
            "直接启动" <- w958
            "启动模块" <- w955
          }
          frame #1 {
            n592 = Bundle By Name(cluster=T6 {"是否启用仪器"=FALSE, "CODMn"={"启动测量模式"={"测量模式"=enum."水样测量"}, "确定按钮"=FALSE}, "启动模块 3"={"氨氮"=FALSE, "总磷"=FALSE, "总氮"=FALSE, "COD"=FALSE}, "常规启动"=FALSE, "直接启动"=FALSE} ("输出簇"), "是否启用仪器"=TRUE, "启动模块 3"=w967, "常规启动"=w966, "直接启动"=w965) -> (w960:T6)
            "输出簇" <- w960
            n593 = vi-ref "质控单元.lvlib:一体站流程质控自动启动.vi"() -> (w963:refnum<vi>)
            n594 = property class="VI"(reference=w963) -> ("Name"=w964:string, "Exec.State"=w962:T16)  [unwired: 1 in, 2 out]
            n595 = case shown="\"Idle\"" w962 {
              tunnel: w964 -> [_ w979]
              tunnel: w960 -> [_ w978]
              frame "Bad", Default {
              }
              frame "Idle" {
                n596 = Open VI Reference(type specifier VI Refnum (for type only)=refnum<vi> refnum ("类型说明符VI引用句柄（仅用于类型）"), vi path=w979, options=128 ("选项")) -> (vi reference=w980:refnum<vi>, error out=w975:errorcluster)  [unwired: 3 in]
                n597 = call-by-ref "开始异步调用"(reference=w980, error in=w975, "CODMn量程切换"="CODMn量程选择", "总磷量程切换"="总磷量程选择", "总氮量程切换"="总氮量程选择", "氨氮量程切换"="氨氮量程选择", "参数"=w978) -> (reference out=w977:refnum<vi>, error out=w976:errorcluster)  [unwired: 7 in]
                n598 = Close Reference(reference=w977, error in (no error)=w976) -> ()  [unwired: 1 out]
              }
            }
          }
        }
      }
      event "报警清除": Value Change {
        w981 = FALSE ("氨氮中断报警")
        n599 = event-data() -> ()  [unwired: 1 in, 6 out]
        n600 = local read "氨氮"() -> (w993:bool)
        n601 = local read "氨氮"() -> (w984:bool)
        n602 = case shown="真" w993 {
          tunnel: [errorcluster {"status"=FALSE, "code"=0, "source"=""} ("error out") w1024] -> w990
          frame False {
          }
          frame True {
            n603 = call "多个线圈写入.vi"("values"=bool[] [TRUE], "starting address"=u16 2106, "Slave ID"=u8 1) -> ("error out"=w1024:errorcluster)  [unwired: 8 in]
          }
        }
        n604 = local read "总磷总氮"() -> (w992:bool)
        n605 = local read "总磷总氮"() -> (w985:bool)
        n606 = case shown="真" w992 {
          tunnel: w990 -> [w1017 w1020]
          tunnel: [w1017 w1018] -> w989
          frame False {
          }
          frame True {
            n607 = call "多个线圈写入.vi"("Error in"=w1020, "values"=bool[] [TRUE], "starting address"=u16 2106, "Slave ID"=u8 2) -> ("error out"=w1018:errorcluster)  [unwired: 7 in]
          }
        }
        n608 = local read "CODMn"() -> (w991:bool)
        n609 = local read "CODMn"() -> (w986:bool)
        n610 = global write "质控中断报警全局.vi" "CODMn中断报警"(w981) -> ()
        n611 = global write "质控中断报警全局.vi" "氨氮中断报警"(w981) -> ()
        n612 = global write "质控中断报警全局.vi" "总氮中断报警"(w981) -> ()
        n613 = global write "质控中断报警全局.vi" "总磷中断报警"(w981) -> ()
        n614 = case shown="真" w991 {
          tunnel: w989 -> [w1011 w1015]
          tunnel: [w1011 w1012] -> w983
          frame False {
          }
          frame True {
            n615 = call "多个线圈写入.vi"("Error in"=w1015, "values"=bool[] [TRUE], "starting address"=u16 2106, "Slave ID"=u8 3) -> ("error out"=w1012:errorcluster)  [unwired: 7 in]
          }
        }
        n616 = case shown="真" w984 {
          tunnel: [w1006 w1007] -> w987
          tunnel: w983 -> [w1006 _]
          frame False {
          }
          frame True {
            n617 = call "多个线圈写入.vi"("values"=bool[] [FALSE], "starting address"=u16 2106, "Slave ID"=u8 1) -> ("error out"=w1007:errorcluster)  [unwired: 8 in]
          }
        }
        n618 = case shown="真" w985 {
          tunnel: w987 -> [w1000 w1003]
          tunnel: [w1000 w1001] -> w988
          frame False {
          }
          frame True {
            n619 = call "多个线圈写入.vi"("Error in"=w1003, "values"=bool[] [FALSE], "starting address"=u16 2106, "Slave ID"=u8 2) -> ("error out"=w1001:errorcluster)  [unwired: 7 in]
          }
        }
        n620 = case shown="真" w986 {
          tunnel: w988 -> [w994 w998]
          tunnel: [w994 w995] -> w982
          frame False {
          }
          frame True {
            n621 = call "多个线圈写入.vi"("Error in"=w998, "values"=bool[] [FALSE], "starting address"=u16 2106, "Slave ID"=u8 3) -> ("error out"=w995:errorcluster)  [unwired: 7 in]
          }
        }
      }
      event "氨氮加标回收启动": Value Change {
        n622 = event-data() -> ()  [unwired: 1 in, 6 out]
        n623 = local read "总磷模块选择"() -> (w1028:enum32{"氨氮总磷", "总氮总磷"})
        n624 = case shown="\"总氮总磷\"" w1028 {
          frame "氨氮总磷", Default {
            w1029 = FALSE ("总氮")
            w1030 = TRUE ("氨氮")
            n625 = call "质控启动参数选择对话框.vi"("COD"=w1029, "总氮"=w1029, "总磷"=w1030, "氨氮"=w1030) -> ("确定启动"=w1032:bool, "启动模块"=w1031:T3)  [unwired: 5 in, 1 out]
            n626 = case shown="真" w1032 {
              tunnel: w1031 -> [_ w1035]
              frame False {
              }
              frame True {
                n627 = vi-ref "氨氮总磷流程质控自动启动.vi"() -> (w1038:refnum<vi>)
                n628 = Unbundle By Name(w1035) -> ("氨氮"=w1034:bool, "总磷"=w1033:bool)
                n629 = property class="VI"(reference=w1038) -> ("Name"=w1036:string, "Exec.State"=w1037:T16)  [unwired: 1 in, 2 out]
                n630 = case shown="\"Idle\"" w1037 {
                  tunnel: w1036 -> [_ w1047 _ _]
                  tunnel: w1034 -> [_ w1041 _ _]
                  tunnel: w1033 -> [_ w1040 _ _]
                  frame "Bad", Default {
                  }
                  frame "Idle" {
                    n631 = Bundle By Name(cluster=T14 {"是否启用仪器"=FALSE, "CODMn"={"启动测量模式"={"测量模式"=enum."水样测量"}, "确定按钮"=FALSE}, "启动模块"={"氨氮"=FALSE, "总磷"=FALSE, "总氮"=FALSE, "COD"=FALSE}, "常规启动"=FALSE, "直接启动"=FALSE} ("参数"), "启动模块.氨氮"=w1041, "启动模块.总磷"=w1040) -> (w1042:T14)
                    n632 = local read "总磷量程选择"() -> (w1039:enum32{"H", "L", "AUTO"})
                    n633 = local read "氨氮量程选择"() -> (w1046:enum32{"H", "L", "AUTO"})
                    n634 = Open VI Reference(type specifier VI Refnum (for type only)=refnum<vi> refnum ("类型说明符VI引用句柄（仅用于类型）"), vi path=w1047, options=128 ("选项")) -> (vi reference=w1051:refnum<vi>, error out=w1045:errorcluster)  [unwired: 3 in]
                    n635 = call-by-ref "开始异步调用"(reference=w1051, error in=w1045, "总磷量程切换"=w1039, "氨氮量程切换"=w1046, "参数"=w1042) -> (reference out=w1050:refnum<vi>, error out=w1044:errorcluster)  [unwired: 9 in]
                    n636 = Close Reference(reference=w1050, error in (no error)=w1044) -> ()  [unwired: 1 out]
                  }
                  frame "Run top level" {
                  }
                  frame "Running" {
                  }
                }
              }
            }
          }
          frame "总氮总磷" {
            n637 = Two Button Dialog(message="确定启动氨氮的加标回收？" ("消息"), 1:"否" ("F按钮名称（“取消”）"), 2:"是" ("T按钮名称（“确定”）")) -> (T button?=w1052:bool)
            n638 = case shown="真" w1052 {
              frame False {
              }
              frame True {
                n639 = vi-ref "质控单元.lvlib:氨氮流程质控自动启动.vi"() -> (w1058:refnum<vi>)
                n640 = property class="VI"(reference=w1058) -> ("Name"=w1056:string, "Exec.State"=w1057:T16)  [unwired: 1 in, 2 out]
                n641 = case shown="\"Idle\"" w1057 {
                  tunnel: w1056 -> [_ w1062 _ _]
                  frame "Bad", Default {
                  }
                  frame "Idle" {
                    n642 = local read "氨氮量程选择"() -> (w1061:enum32{"H", "L", "AUTO"})
                    n643 = Open VI Reference(type specifier VI Refnum (for type only)=refnum<vi> refnum ("类型说明符VI引用句柄（仅用于类型）"), vi path=w1062, options=128 ("选项")) -> (vi reference=w1066:refnum<vi>, error out=w1060:errorcluster)  [unwired: 3 in]
                    n644 = call-by-ref "开始异步调用"(reference=w1066, error in=w1060, "氨氮量程切换"=w1061) -> (reference out=w1065:refnum<vi>, error out=w1059:errorcluster)  [unwired: 11 in]
                    n645 = Close Reference(reference=w1065, error in (no error)=w1059) -> ()  [unwired: 1 out]
                  }
                  frame "Run top level" {
                  }
                  frame "Running" {
                  }
                }
              }
            }
          }
        }
      }
      event "总磷总氮加标回收启动": Value Change {
        n646 = event-data() -> ()  [unwired: 1 in, 6 out]
        n647 = local read "总磷模块选择"() -> (w1067:enum32{"氨氮总磷", "总氮总磷"})
        n648 = case shown="\"总氮总磷\"" w1067 {
          frame "氨氮总磷", Default {
            n649 = One Button Dialog(message="请启动氨氮总磷的加标回收！" ("消息")) -> ()  [unwired: 1 in, 1 out]
          }
          frame "总氮总磷" {
            w1071 = TRUE ("总氮")
            w1072 = FALSE ("氨氮")
            n650 = call "质控启动参数选择对话框.vi"("COD"=w1072, "总氮"=w1071, "总磷"=w1071, "氨氮"=w1072) -> ("确定启动"=w1070:bool, "启动模块"=w1069:T3)  [unwired: 5 in, 1 out]
            n651 = case shown="真" w1070 {
              tunnel: w1069 -> [_ w1076]
              frame False {
              }
              frame True {
                n652 = vi-ref "质控单元.lvlib:总磷总氮流程质控自动启动.vi"() -> (w1073:refnum<vi>)
                n653 = Unbundle By Name(w1076) -> ("总磷"=w1075:bool, "总氮"=w1074:bool)
                n654 = property class="VI"(reference=w1073) -> ("Name"=w1077:string, "Exec.State"=w1078:T16)  [unwired: 1 in, 2 out]
                n655 = case shown="\"Idle\"" w1078 {
                  tunnel: w1077 -> [_ w1087 _ _]
                  tunnel: w1075 -> [_ w1080 _ _]
                  tunnel: w1074 -> [_ w1079 _ _]
                  frame "Bad", Default {
                  }
                  frame "Idle" {
                    n656 = Bundle By Name(cluster=T14 {"是否启用仪器"=FALSE, "CODMn"={"启动测量模式"={"测量模式"=enum."水样测量"}, "确定按钮"=FALSE}, "启动模块"={"氨氮"=FALSE, "总磷"=FALSE, "总氮"=FALSE, "COD"=FALSE}, "常规启动"=FALSE, "直接启动"=FALSE} ("参数"), "启动模块.总磷"=w1080, "启动模块.总氮"=w1079) -> (w1081:T14)
                    n657 = local read "总氮量程选择"() -> (w1084:enum32{"H", "L", "AUTO"})
                    n658 = local read "总磷量程选择"() -> (w1083:enum32{"H", "L", "AUTO"})
                    n659 = Open VI Reference(type specifier VI Refnum (for type only)=refnum<vi> refnum ("类型说明符VI引用句柄（仅用于类型）"), vi path=w1087, options=128 ("选项")) -> (vi reference=w1091:refnum<vi>, error out=w1085:errorcluster)  [unwired: 3 in]
                    n660 = call-by-ref "开始异步调用"(reference=w1091, error in=w1085, "总磷量程切换"=w1083, "总氮量程切换"=w1084, "参数"=w1081) -> (reference out=w1090:refnum<vi>, error out=w1086:errorcluster)  [unwired: 9 in]
                    n661 = Close Reference(reference=w1090, error in (no error)=w1086) -> ()  [unwired: 1 out]
                  }
                  frame "Run top level" {
                  }
                  frame "Running" {
                  }
                }
              }
            }
          }
        }
      }
      event "CODMn加标回收启动": Value Change {
        n662 = event-data() -> ()  [unwired: 1 in, 6 out]
        n663 = Two Button Dialog(message="确定启动CODMn的加标回收？" ("消息"), 1:"否" ("F按钮名称（“取消”）"), 2:"是" ("T按钮名称（“确定”）")) -> (T button?=w1092:bool)
        n664 = case shown="真" w1092 {
          frame False {
          }
          frame True {
            n665 = vi-ref "质控单元.lvlib:CODMn流程质控自动启动.vi"() -> (w1098:refnum<vi>)
            n666 = property class="VI"(reference=w1098) -> ("Name"=w1096:string, "Exec.State"=w1097:T16)  [unwired: 1 in, 2 out]
            n667 = case shown="\"Idle\"" w1097 {
              tunnel: w1096 -> [_ w1102 _ _]
              frame "Bad", Default {
              }
              frame "Idle" {
                n668 = local read "CODMn量程选择"() -> (w1099:enum32{"H", "L", "AUTO"})
                n669 = Open VI Reference(type specifier VI Refnum (for type only)=refnum<vi> refnum ("类型说明符VI引用句柄（仅用于类型）"), vi path=w1102, options=128 ("选项")) -> (vi reference=w1106:refnum<vi>, error out=w1101:errorcluster)  [unwired: 3 in]
                n670 = call-by-ref "开始异步调用"(reference=w1106, error in=w1101, "CODMn量程切换"=w1099) -> (reference out=w1105:refnum<vi>, error out=w1100:errorcluster)  [unwired: 10 in]
                n671 = Close Reference(reference=w1105, error in (no error)=w1100) -> ()  [unwired: 1 out]
              }
              frame "Run top level" {
              }
              frame "Running" {
              }
            }
          }
        }
      }
      event "平行样测试": Value Change {
        n672 = event-data() -> ()  [unwired: 1 in, 6 out]
        n673 = flat-sequence {
          tunnel: [w1112] -> w1110
          tunnel: [w1114] -> w1109
          tunnel: [w1113] -> w1108
          tunnel: w1107 -> [w1111]
          tunnel: w1110 -> [w1121]
          tunnel: w1109 -> [w1120]
          tunnel: w1108 -> [w1119]
          frame #0 {
            n674 = Cancel Notification(0:w1111) -> ()  [unwired: 1 in, 3 out]
            n675 = call "平行样启动流程对话框.vi"() -> ("启动模块"=w1112:cluster{"氨氮1":bool, "总磷1":bool, " COD1":bool}, "直接启动"=w1113:bool, "常规启动"=w1114:bool)  [unwired: 8 in, 1 out]
            "常规启动 2" <- w1114
            "直接启动 2" <- w1113
            "启动模块 2" <- w1112
          }
          frame #1 {
            n676 = Bundle By Name(cluster=T5 {"是否启用仪器"=FALSE, "CODMn"={"启动测量模式"={"测量模式"=enum."水样测量"}, "确定按钮"=TRUE}, "启动模块"={"氨氮1"=FALSE, "总磷1"=FALSE, " COD1"=FALSE}, "常规启动"=FALSE, "直接启动"=FALSE} ("参数"), "是否启用仪器"=TRUE, "启动模块"=w1121, "常规启动"=w1120, "直接启动"=w1119) -> (w1116:T5)
            "输出簇 2" <- w1116
            n677 = vi-ref "一体站流程平行样自动启动.vi"() -> (w1117:refnum<vi>)
            n678 = property class="VI"(reference=w1117) -> ("Name"=w1118:string, "Exec.State"=w1115:T16)  [unwired: 1 in, 2 out]
            n679 = case shown="\"Idle\"" w1115 {
              tunnel: w1118 -> [_ w1130]
              tunnel: w1116 -> [_ w1124]
              frame "Bad", Default {
              }
              frame "Idle" {
                n680 = Open VI Reference(type specifier VI Refnum (for type only)=refnum<vi> refnum ("类型说明符VI引用句柄（仅用于类型）"), vi path=w1130, options=128 ("选项")) -> (vi reference=w1131:refnum<vi>, error out=w1129:errorcluster)  [unwired: 3 in]
                n681 = call-by-ref "开始异步调用"(reference=w1131, error in=w1129, "参数"=w1124) -> (reference out=w1126:refnum<vi>, error out=w1125:errorcluster)  [unwired: 9 in]
                n682 = Close Reference(reference=w1126, error in (no error)=w1125) -> ()  [unwired: 1 out]
              }
            }
          }
        }
      }
      event "停止测量": Value Change {
        w1132 = TRUE ("氨氮")
        # "停止采配水、氨氮、总磷总氮、COD、质控"
        n683 = event-data() -> ()  [unwired: 1 in, 6 out]
        n684 = call "质控启动参数选择对话框.vi"("COD"=w1132, "总氮"=w1132, "总磷"=w1132, "氨氮"=w1132) -> ("确定启动"=w1133:bool, "启动模块"=w1134:T3)  [unwired: 5 in, 1 out]
        n685 = case shown="真" w1133 {
          tunnel: w1134 -> [_ w1144]
          frame False {
          }
          frame True {
            n686 = Unbundle By Name(w1144) -> ("氨氮"=w1142:bool, "总磷"=w1141:bool, "总氮"=w1140:bool, "COD"=w1143:bool)
            n687 = Or(x=w1141, y=w1140) -> (x .or. y?=w1139:bool)
            n688 = case shown="真" w1143 {
              frame False {
              }
              frame True {
                n689 = call "CODMn停止命令 (子VI).vi"() -> ()  [unwired: 12 in]
                n690 = Obtain Notifier(name (unnamed)="CODMn" ("名称（未命名）"), notification data type=FALSE) -> (notifier out=w1170:refnum<notifier>)  [unwired: 2 in, 2 out]
                n691 = Send Notification(notification=TRUE ("通知"), notifier=w1170) -> ()  [unwired: 1 in, 2 out]
                n692 = call "单个写入.vi"("value"=u16 2, "address"=u16 103, "Slave ID"=u8 3) -> ()  [unwired: 8 in, 1 out]
              }
            }
            n693 = case shown="真" w1142 {
              frame False {
              }
              frame True {
                n694 = Obtain Queue(name (unnamed)="NH3N" ("名称（未命名）"), element data type=cluster{"命令":string, "data":variant} {"命令"="", "data"=variant}) -> (queue out=w1166:refnum<queue>)  [unwired: 3 in, 2 out]
                n695 = Enqueue Element(queue=w1166, element=cluster{"命令":string, "data":variant} {"命令"="启动", "data"=variant(cluster{"站号":u16, "控制命令输出":u16[]} {"站号"=1, "控制命令输出"=[2816]})} ("元素")) -> ()  [unwired: 2 in, 3 out]
                n696 = Obtain Notifier(name (unnamed)="NH3N" ("名称（未命名）"), notification data type=FALSE) -> (notifier out=w1162:refnum<notifier>)  [unwired: 2 in, 2 out]
                n697 = Send Notification(notification=TRUE ("通知"), notifier=w1162) -> ()  [unwired: 1 in, 2 out]
                n698 = call "单个写入.vi"("value"=u16 2, "address"=u16 103, "Slave ID"=u8 1) -> ()  [unwired: 8 in, 1 out]
              }
            }
            n699 = case shown="真" w1139 {
              frame False {
              }
              frame True {
                n700 = Obtain Queue(name (unnamed)="TP" ("名称（未命名）"), element data type=cluster{"命令":string, "data":variant} {"命令"="", "data"=variant}) -> (queue out=w1155:refnum<queue>)  [unwired: 3 in, 2 out]
                n701 = Enqueue Element(queue=w1155, element=cluster{"命令":string, "data":variant} {"命令"="启动", "data"=variant(cluster{"站号":u16, "控制命令输出":u16[]} {"站号"=1, "控制命令输出"=[2816]})} ("元素")) -> ()  [unwired: 2 in, 3 out]
                n702 = Obtain Notifier(name (unnamed)="TNTP" ("名称（未命名）"), notification data type=FALSE) -> (notifier out=w1151:refnum<notifier>)  [unwired: 2 in, 2 out]
                n703 = Send Notification(notification=TRUE ("通知"), notifier=w1151) -> ()  [unwired: 1 in, 2 out]
                n704 = call "单个写入.vi"("value"=u16 2, "address"=u16 103, "Slave ID"=u8 2) -> ()  [unwired: 8 in, 1 out]
              }
            }
          }
        }
        n705 = Send Notification(notification=TRUE ("通知"), notifier=w1138) -> ()  [unwired: 1 in, 2 out]
        n706 = Enqueue Element At Opposite End(queue=w1135, element=T15 {"命令"="单个写入", {"starting address"=300, "holding register value"=2}} ("元素")) -> ()  [unwired: 2 in, 3 out]
      }
      event "查看": Value Change {
        n707 = event-data() -> ()  [unwired: 1 in, 6 out]
        n708 = property on="窗格" class="Pane"("Origin"=T7 {"Horizontal"=0, "Vertical"=600} ("原点")) -> ()  [unwired: 2 in, 2 out]
      }
      event "返回": Value Change {
        n709 = event-data() -> ()  [unwired: 1 in, 6 out]
        n710 = property on="窗格" class="Pane"("Origin"=T7 {"Horizontal"=0, "Vertical"=0} ("原点")) -> ()  [unwired: 2 in, 2 out]
      }
    }
  }
  n711 = Build Array("时间" ("table"), "参数" ("table"), "加标前水样测试时间" ("table"), "加标前水样浓度值" ("元素"), "加标后水样浓度值" ("元素"), "加标母液浓度值" ("元素"), "加标体积" ("元素"), "加标水杯定容体积" ("元素"), "加标回收率" ("元素")) -> (→"columns":string[])
  n712 = local write "背隙补偿步数 2"(w89) -> ()
  n713 = call-poly <vilib>:"Read Key.vi"("section"=w96, "error in (no error)"=w91, "key"="背隙值3", "refnum"=w92) -> ("error out"=w85:errorcluster, "value"=w87:i32, "refnum out"=w86:T13)  [unwired: 4 in, 1 out]
  n714 = local write "背隙补偿步数 3"(w87) -> ()
  n715 = call-poly <vilib>:"Read Key.vi"("section"=w78, "error in (no error)"=w85, "key"="标准体积1", "refnum"=w86) -> ("error out"=w81:errorcluster, "value"=w83:dbl, "refnum out"=w82:T13)  [unwired: 4 in, 1 out]
  n716 = local write "标准体积 1"(w83) -> ()
  n717 = call-poly <vilib>:"Read Key.vi"("section"=w78, "error in (no error)"=w81, "key"="标准体积2", "refnum"=w82) -> ("error out"=w79:errorcluster, "value"=w72:dbl, "refnum out"=w80:T13)  [unwired: 4 in, 1 out]
  n718 = local write "标准体积 2"(w72) -> ()
  n719 = call-poly <vilib>:"Read Key.vi"("section"=w78, "error in (no error)"=w79, "key"="标准体积3", "refnum"=w80) -> ("error out"=w76:errorcluster, "value"=w71:dbl, "refnum out"=w77:T13)  [unwired: 4 in, 1 out]
  n720 = local write "标准体积 3"(w71) -> ()
  n721 = call-poly <vilib>:"Read Key.vi"("section"=w78, "error in (no error)"=w76, "key"="标准体积4", "refnum"=w77) -> ("error out"=w74:errorcluster, "value"=w56:dbl, "refnum out"=w75:T13)  [unwired: 4 in, 1 out]
  n722 = local write "标准体积 4"(w56) -> ()
  n723 = call-poly <vilib>:"Read Key.vi"("section"=w78, "error in (no error)"=w74, "key"="标准体积5", "refnum"=w75) -> ("error out"=w65:errorcluster, "value"=w55:dbl, "refnum out"=w66:T13)  [unwired: 4 in, 1 out]
  n724 = local write "标准体积 5"(w55) -> ()
  n725 = call-poly <vilib>:"Read Key.vi"("section"=w78, "error in (no error)"=w65, "key"="实际体积1", "refnum"=w66) -> ("error out"=w63:errorcluster, "value"=w54:dbl, "refnum out"=w64:T13)  [unwired: 4 in, 1 out]
  n726 = local write "实际体积 1"(w54) -> ()
  n727 = call-poly <vilib>:"Read Key.vi"("section"=w78, "error in (no error)"=w63, "key"="实际体积2", "refnum"=w64) -> ("error out"=w61:errorcluster, "value"=w53:dbl, "refnum out"=w62:T13)  [unwired: 4 in, 1 out]
  n728 = local write "实际体积 2"(w53) -> ()
  n729 = call-poly <vilib>:"Read Key.vi"("section"=w78, "error in (no error)"=w61, "key"="实际体积3", "refnum"=w62) -> ("error out"=w59:errorcluster, "value"=w50:dbl, "refnum out"=w60:T13)  [unwired: 4 in, 1 out]
  n730 = local write "实际体积 3"(w50) -> ()
  n731 = call-poly <vilib>:"Read Key.vi"("section"=w78, "error in (no error)"=w59, "key"="实际体积4", "refnum"=w60) -> ("error out"=w57:errorcluster, "value"=w49:dbl, "refnum out"=w58:T13)  [unwired: 4 in, 1 out]
  n732 = call-dynamic "Close Session.vi"("error in (no error)"=w144, "MB_Serial session"=w104) -> ()  [unwired: 9 in, 1 out]
  n733 = local write "实际体积 4"(w49) -> ()
  n734 = call-poly <vilib>:"Read Key.vi"("section"=w78, "error in (no error)"=w57, "key"="实际体积5", "refnum"=w58) -> ("error out"=w44:errorcluster, "value"=w48:dbl, "refnum out"=w45:T13)  [unwired: 4 in, 1 out]
  n735 = local write "实际体积 5"(w48) -> ()
  n736 = call-poly <vilib>:"Read Key.vi"("section"="质控手动体积选择", "error in (no error)"=w44, "key"="手动体积选择" ("section"), "refnum"=w45) -> ("error out"=w39:errorcluster, "value"=w41:i32, "refnum out"=w40:T13)  [unwired: 4 in, 1 out]
  n737 = local write "注出体积选择"(w41) -> ()
  n738 = call-poly <vilib>:"Read Key.vi"("section"=w7, "error in (no error)"=w39, "key"="模块1" ("section"), "refnum"=w40) -> ("error out"=w37:errorcluster, "value"=w29:bool, "refnum out"=w38:T13)  [unwired: 4 in, 1 out]
  n739 = call-poly <vilib>:"Read Key.vi"("section"=w7, "error in (no error)"=w37, "key"="模块2" ("section"), "refnum"=w38) -> ("error out"=w35:errorcluster, "value"=w30:bool, "refnum out"=w36:T13)  [unwired: 4 in, 1 out]
  n740 = local write "氨氮"(w29) -> ()
  n741 = local write "总磷总氮"(w30) -> ()
  n742 = call-poly <vilib>:"Read Key.vi"("section"=w7, "error in (no error)"=w35, "key"="模块3" ("section"), "refnum"=w36) -> ("error out"=w10:errorcluster, "value"=w31:bool, "refnum out"=w11:T13)  [unwired: 4 in, 1 out]
  n743 = local write "CODMn"(w31) -> ()
  n744 = call-poly <vilib>:"Read Key.vi"("section"=w7, "error in (no error)"=w10, "key"="总磷模块" ("section"), "refnum"=w11) -> ("error out"=w8:errorcluster, "value"=w5:i32, "refnum out"=w9:T13)  [unwired: 4 in, 1 out]
  n745 = local write "总磷模块选择"(w5) -> ()
  n746 = global write "质控测完标志全局 1.vi" "总磷模块选择"(w5) -> ()
  n747 = call-poly <vilib>:"Read Key.vi"("section"=w28, "error in (no error)"=w8, "key"="氨氮" ("section"), "refnum"=w9) -> ("error out"=w26:errorcluster, "value"=w15:u32, "refnum out"=w27:T13)  [unwired: 4 in, 1 out]
  n748 = local write "氨氮量程选择"(w15) -> ()
  n749 = call-poly <vilib>:"Read Key.vi"("section"=w28, "error in (no error)"=w26, "key"="总氮" ("section"), "refnum"=w27) -> ("error out"=w24:errorcluster, "value"=w14:u32, "refnum out"=w25:T13)  [unwired: 4 in, 1 out]
  n750 = local write "总氮量程选择"(w14) -> ()
  n751 = call-poly <vilib>:"Read Key.vi"("section"=w28, "error in (no error)"=w24, "key"="总磷" ("section"), "refnum"=w25) -> ("error out"=w22:errorcluster, "value"=w13:u32, "refnum out"=w23:T13)  [unwired: 4 in, 1 out]
  n752 = local write "总磷量程选择"(w13) -> ()
  n753 = call-poly <vilib>:"Read Key.vi"("section"=w28, "error in (no error)"=w22, "key"="CODMn" ("section"), "refnum"=w23) -> ("error out"=w20:errorcluster, "value"=w12:u32, "refnum out"=w21:T13)  [unwired: 4 in, 1 out]
  n754 = local write "CODMn量程选择"(w12) -> ()
  n755 = call <vilib>:"Close Config Data.vi"("error in (no error)"=w20, "refnum"=w21) -> ()  [unwired: 8 in, 2 out]
  "VISA Resource" <- w4
  "Serial Config" <- w103
  "COM口" <- w4
